vi "multi-rev.vi"(11 "设备信息":T2) -> ()   [LabVIEW 2020]
uses:
  <vilib>/Utility/NIReport.llb/Report Type.ctl
  <vilib>/Utility/NIReport.llb/Append Numeric Table to Report (wrap).vi
  <vilib>/Utility/NIReport.llb/Append Text Table to Report (wrap).vi
  <vilib>/Utility/NIReport.llb/NI_report.lvclass
  support/Message Queue/Message Queue.lvlib
  support/User Event - Stop/User Event - Stop.lvlib
  setup/support/rev_setup.lvlib
  rev_meas/rev_meas.lvlib
  bas_meas/bas_meas.lvlib
  <vilib>/Utility/NIReport.llb/NI_ReportGenerationCore.lvlib
panel:
  in  "新的测量":T1
  in  "calibration":T3
  in  "HWsetup":T4
  in  "EM设置":T5
  in  "开始":T6
  in  "停止":T7
  in  "退出":T8
  in  "测试类型":enum32{"空场当前结果", "放样后当前结果", "分析结果", "导出报告"}(radio)
  out "鼠标抓取值3":T9
  in  "选项卡控件":T10(tab)
  out "鼠标抓取值1":T9
  out "每通道声级":cluster{"声级大小":string, "dB":string}[](array[cluster])
  out "空场测量状态":T11
  in  "空场测试完成状态":T12
  in  "空场测试结果":T13
  out "空场混响频谱图":cluster{dbl[], "所有X坐标":dbl[]}[](graph)
  in  "saveT1":T14
  in  "空场当前结果":i32(listbox)
  in  "T1计数":u32
  in  "loadT1":bool
  in  "空场结果至Excel":bool
  in  "返回空场测试":bool
  in  "deletelineT1":bool
  in  "clearlistT1":bool
  in  "空场测试结果（T1）":i32(listbox)
  out "鼠标抓取值2":T9
  out "放样后每通道声级":cluster{"声级大小":string, "dB":string}[](array[cluster])
  out "放样后测量状态":T11
  in  "放样后测试完成状态":T12
  in  "放样后测试结果":T13
  in  "放入样品后当前结果":i32(listbox)
  out "放入样品后混响频谱图":cluster{dbl[], "所有X坐标":dbl[]}[](graph)
  in  "saveT2":T14
  in  "返回放样后测试":bool
  in  "放入样品后测试结果（T2）":i32(listbox)
  in  "clearlistT2":bool
  in  "deletelineT2":bool
  in  "放样结果至Excel":bool
  in  "loadT2":bool
  in  "T2计数":u32
  in  "ExportReport":T15
  in  "All results to Excel":T16
  out "吸声频谱图":cluster{dbl[], "所有X坐标":dbl[]}[](graph)
  in  "All results":i32(listbox)
  in  "analysis":T17
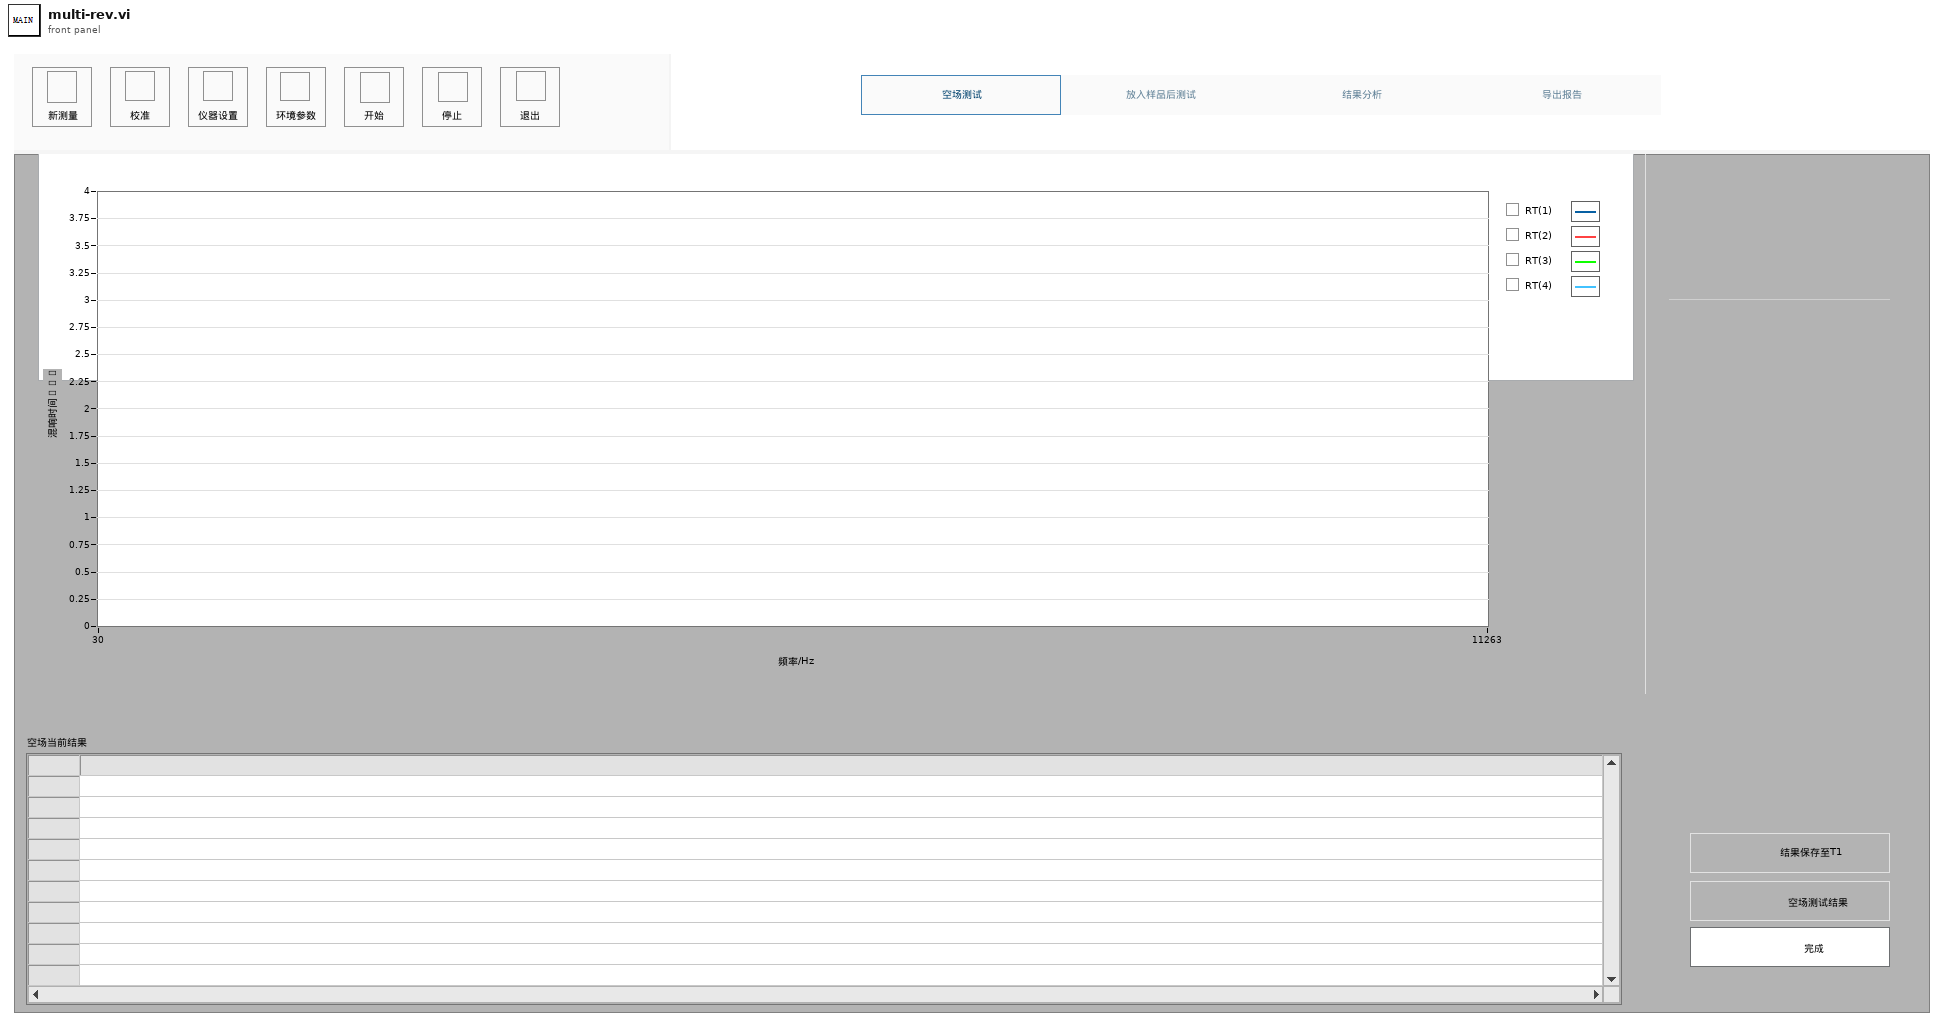
[diagram p1: front panel]
types:
  T1 = typedef "新测量.ctl" = bool
  T2 = cluster{"勾选的设备":refnum<visa-resource-name>[], "设备启用状态":cluster{"通道0":bool, "通道1":bool, "通道2":bool, "通道3":bool}}
  T3 = typedef "校准2.ctl" = bool
  T4 = typedef "硬件设置.ctl" = bool
  T5 = typedef "环境参数设置.ctl" = bool
  T6 = typedef "开始按钮.ctl" = bool
  T7 = typedef "停止按钮.ctl" = bool
  T8 = typedef "停止按钮2.ctl" = bool
  T9 = typedef "图谱移动字符串.ctl" = string
  T10 = enum32{"空场当前结果", "空场测试结果", "放入样品后当前结果", "放入样品后测试结果", "分析结果"}
  T11 = typedef "通道测量状态.ctl" = cluster{"通道编号":string, "通道测量状态":string}[]
  T12 = typedef "完成.ctl" = bool
  T13 = typedef "查看数据.ctl" = bool
  T14 = typedef "结果保存.ctl" = bool
  T15 = typedef "导出报表.ctl" = bool
  T16 = typedef "发送至Excel.ctl" = bool
  T17 = typedef "分析.ctl" = bool
  T18 = cluster{"通道编号输出":u32, "EDT":string, "T20":string, "T30":string}[]
  T19 = cluster{"空场当前结果":refnum<vi>, "放样后当前结果":refnum<vi>, "分析结果":refnum<vi>, "导出报告":refnum<vi>}
  T20 = typedef "Message Queue.lvlib/All Message Queues.ctl" = cluster{"UI":refnum<queue>, "采集":refnum<queue>, "记录":refnum<queue>}
  T21 = cluster{"T1":dbl[], "T2":dbl[], "A1":dbl[], "A2":dbl[], "AT":dbl[], "Aobj":dbl[], "αs":dbl[]}
  T22 = typedef "NI_ReportGenerationCore.lvlib/Report Type.ctl" = enum16{"HTML", "Word", "Excel"}
  T23 = cluster{"position (Excel)":cluster{"row":i32, "column":i32}, "name (Excel)":string, "bookmark (Word)":string}
  T24 = cluster{"T1":string[], "T2":string[], "A1":string[], "A2":string[], "AT":string[], "Aobj":string[], "αs":string[]}
  T25 = enum8{"Enabled", "Disabled", "Disabled and Grayed Out"}
  T26 = typedef "LVPoint32TypeDef.ctl" = cluster{"Horizontal":i32, "Vertical":i32}
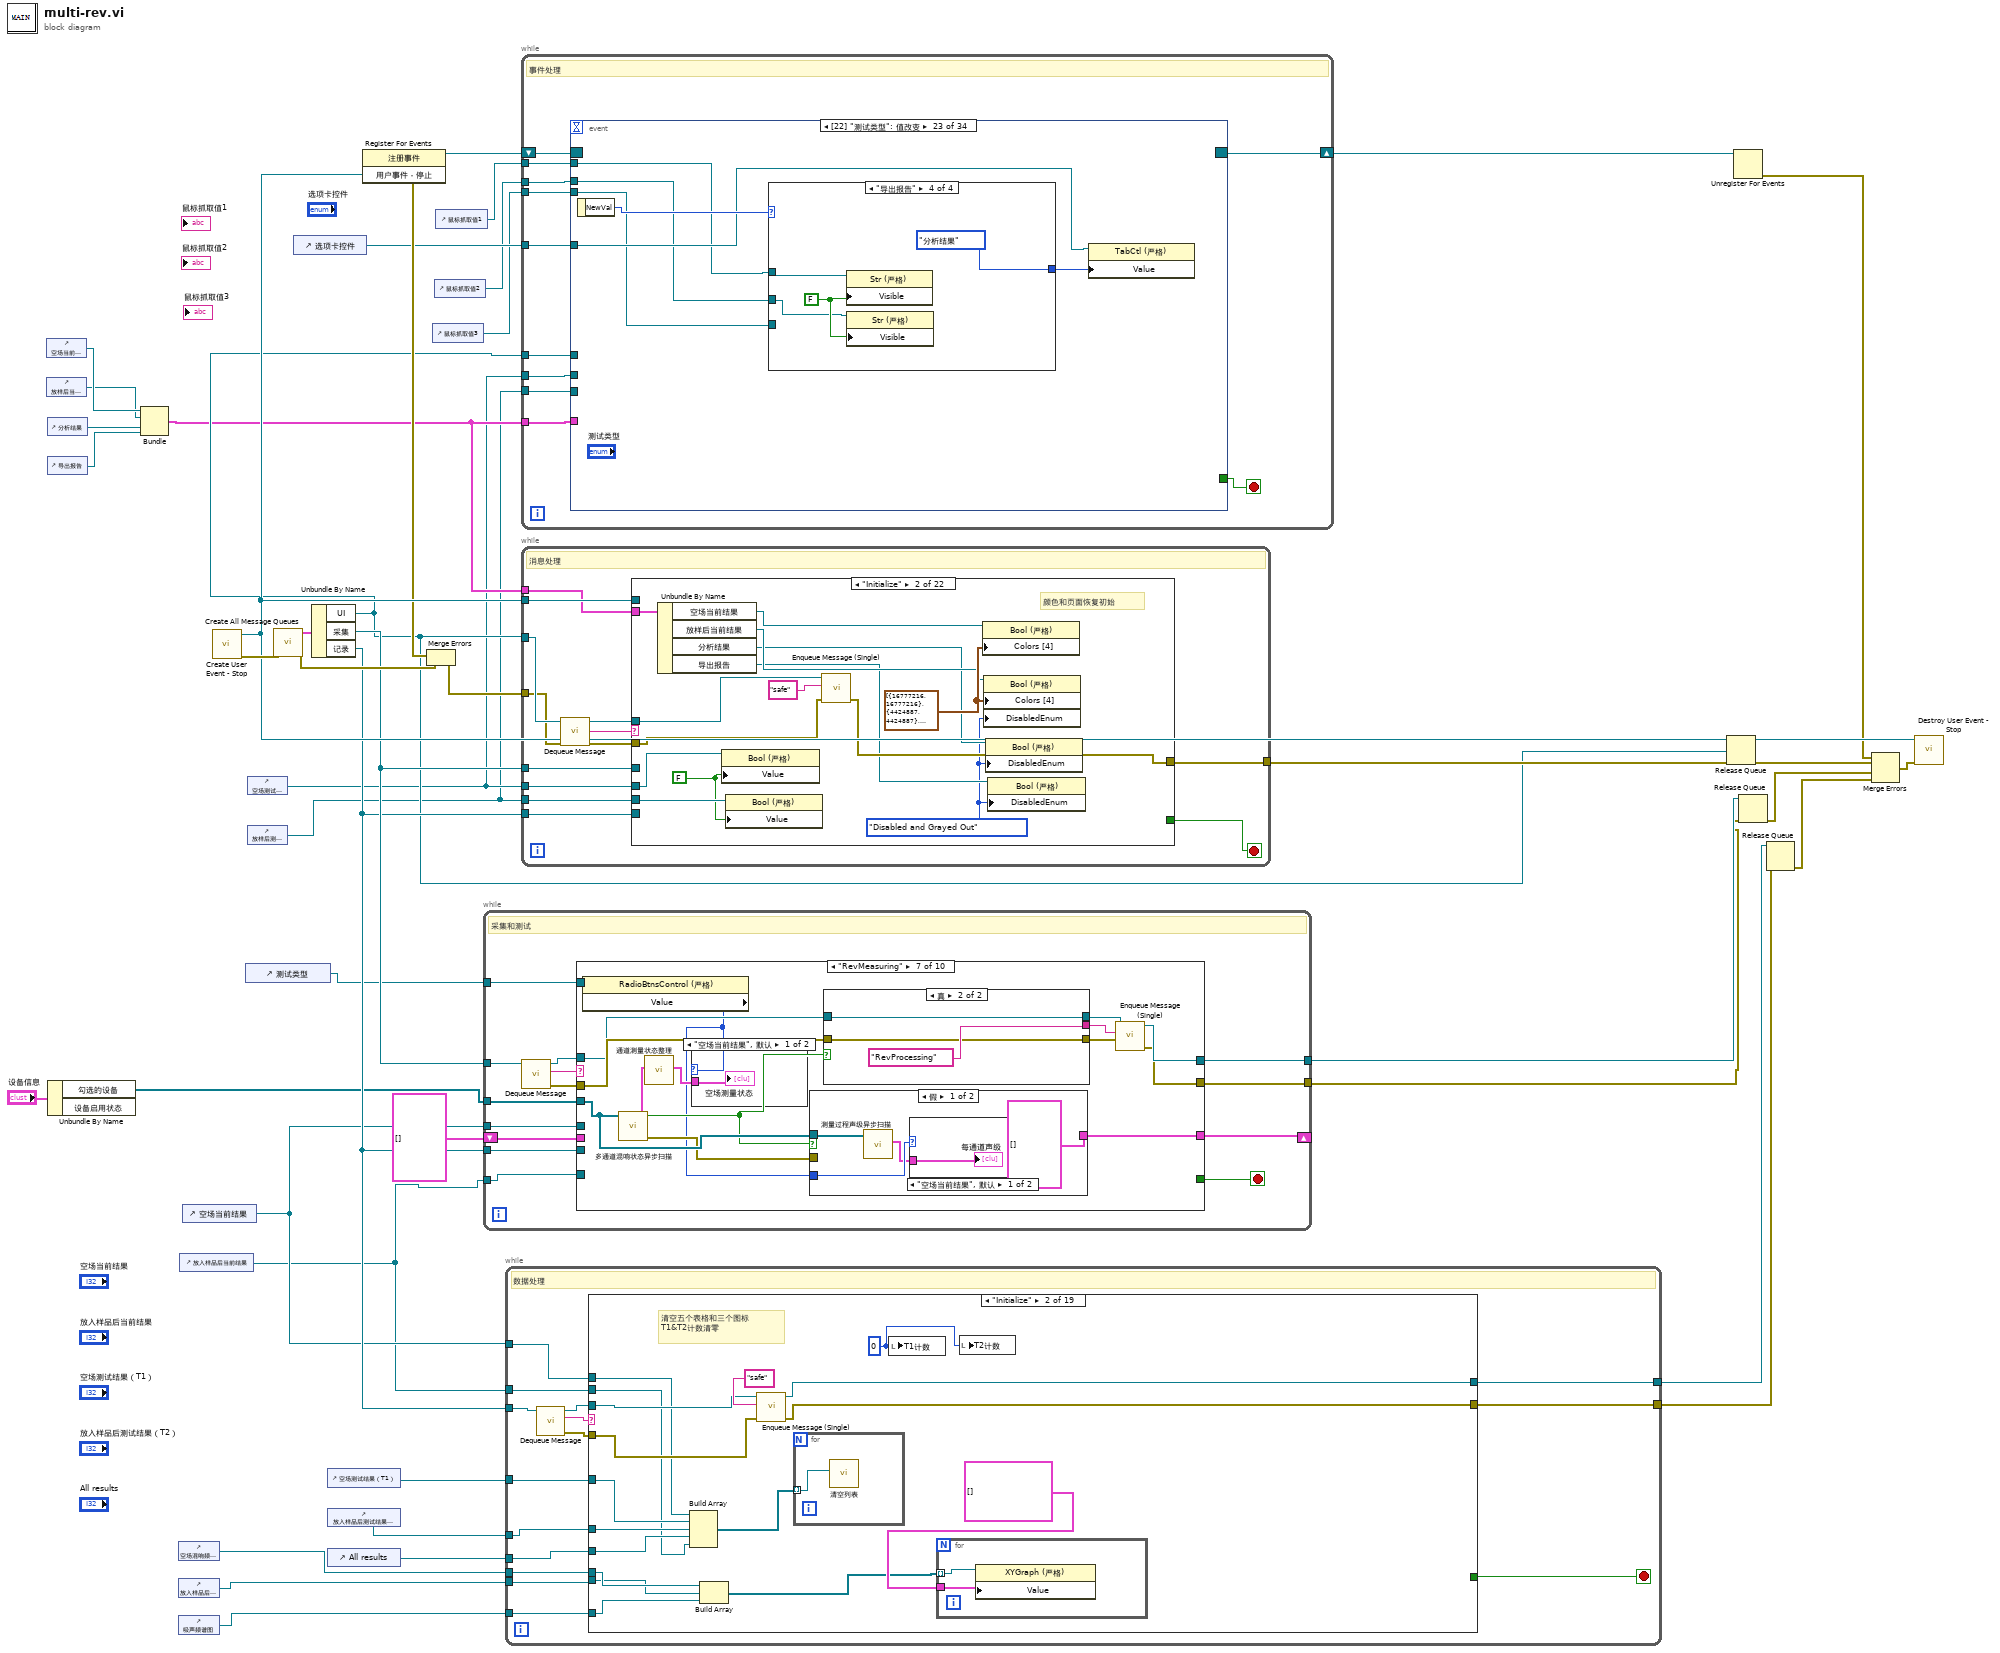
[diagram p0: block diagram]
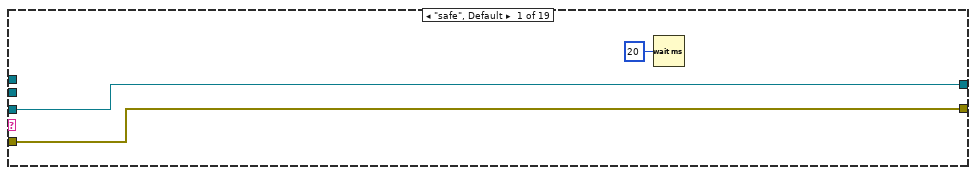
[diagram p2: hidden frame]
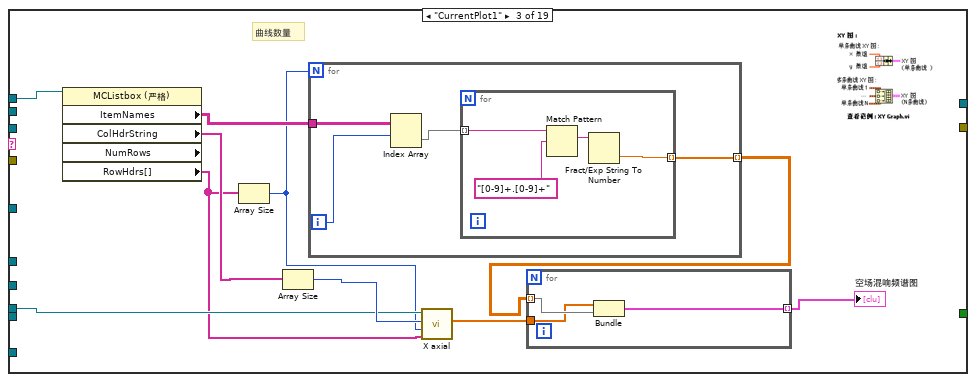
[diagram p3: hidden frame]
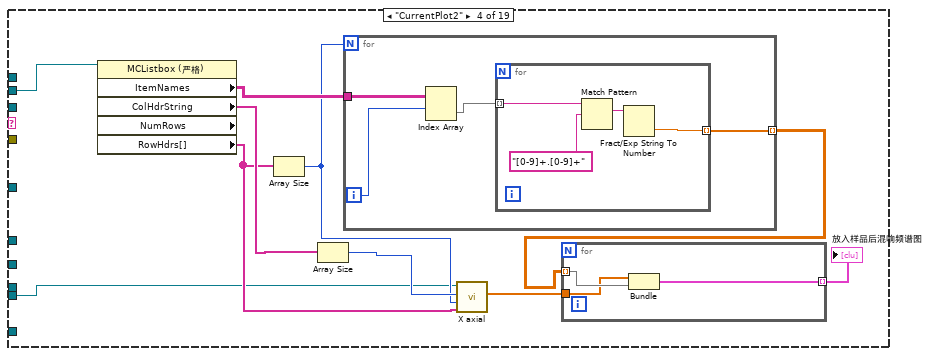
[diagram p4: hidden frame]
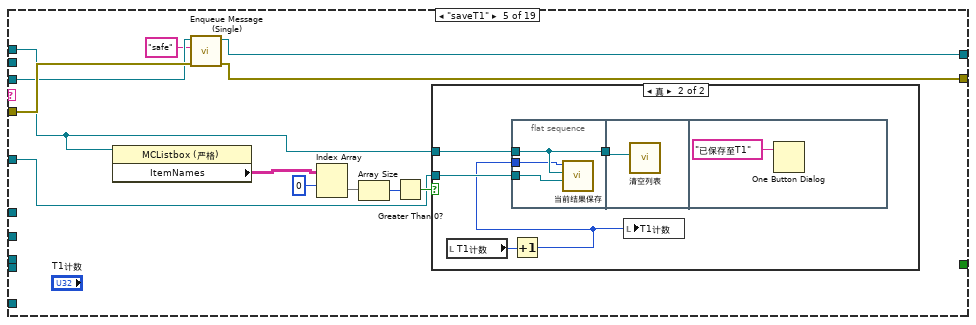
[diagram p5: hidden frame]
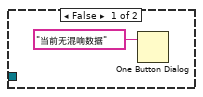
[diagram p6: hidden frame]
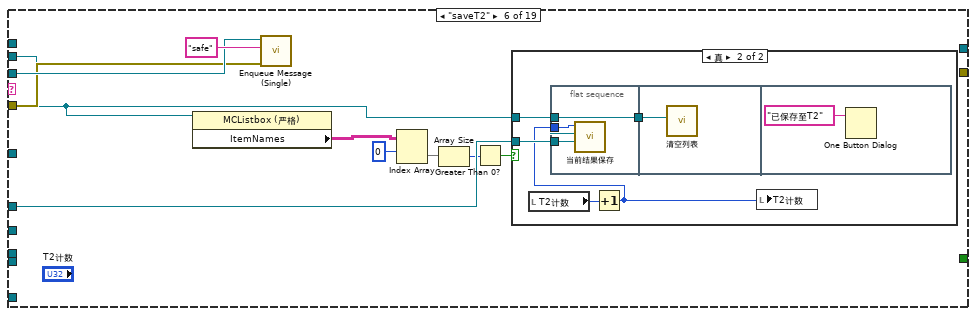
[diagram p7: hidden frame]
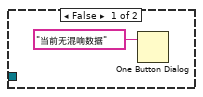
[diagram p8: hidden frame]
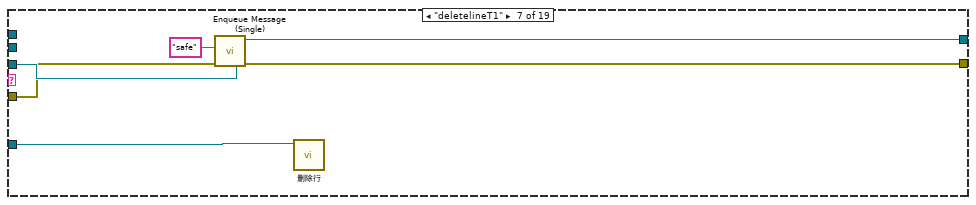
[diagram p9: hidden frame]
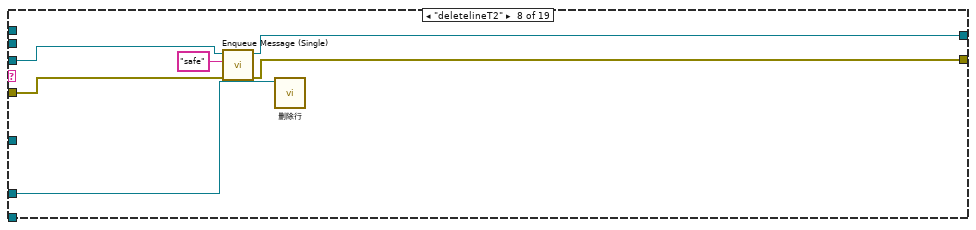
[diagram p10: hidden frame]
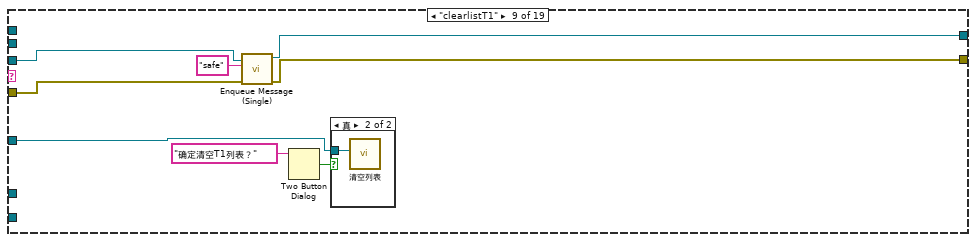
[diagram p11: hidden frame]
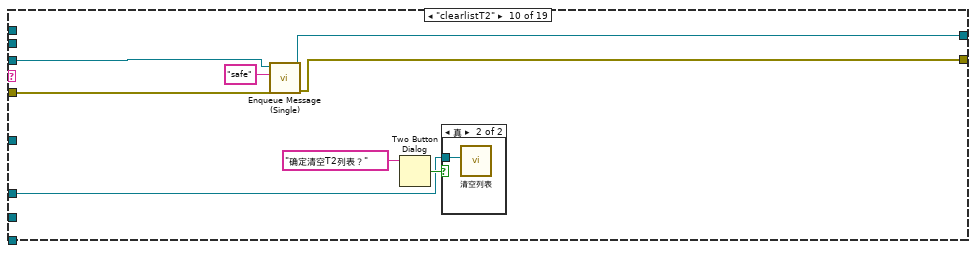
[diagram p13: hidden frame]
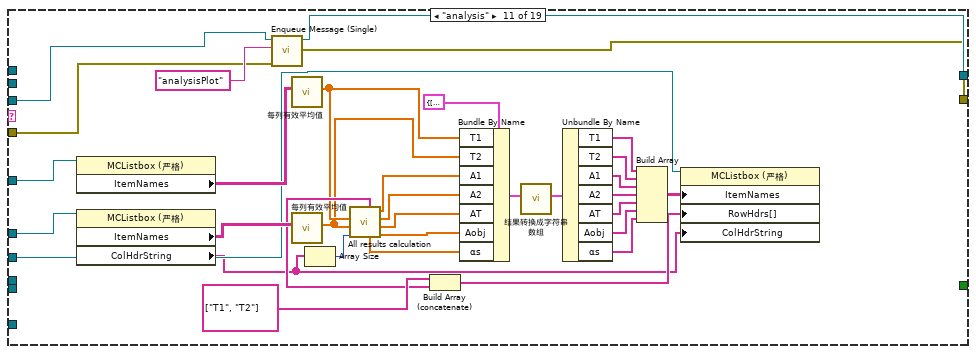
[diagram p15: hidden frame]
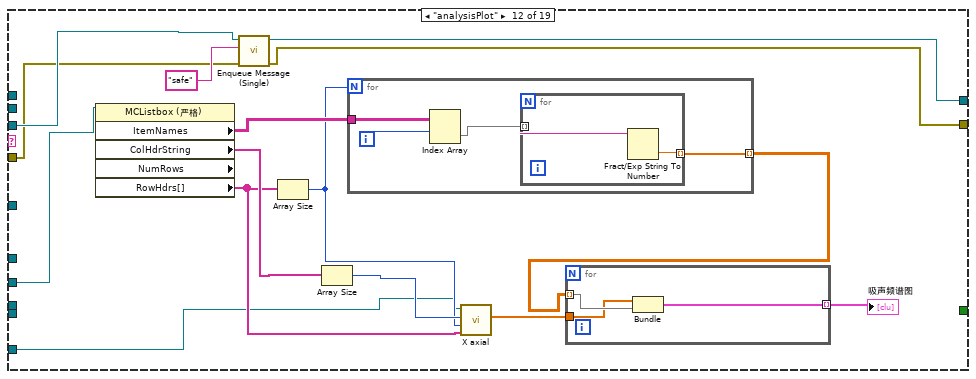
[diagram p16: hidden frame]
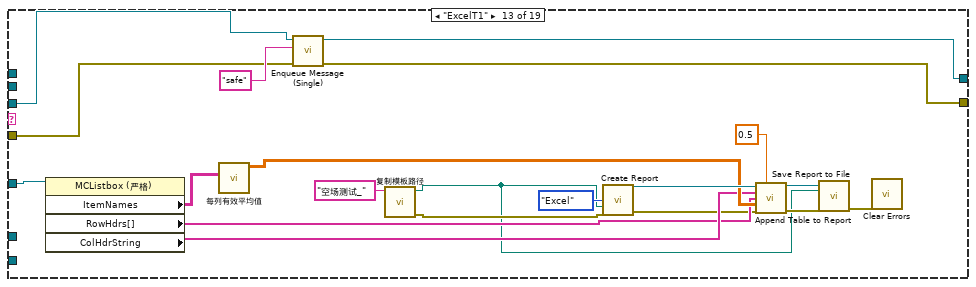
[diagram p17: hidden frame]
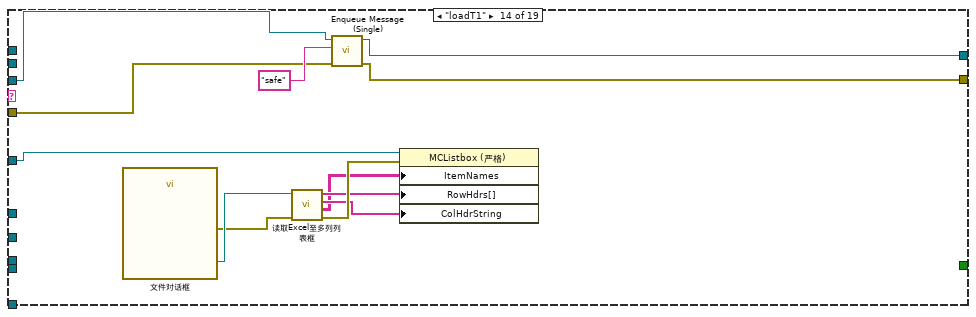
[diagram p18: hidden frame]
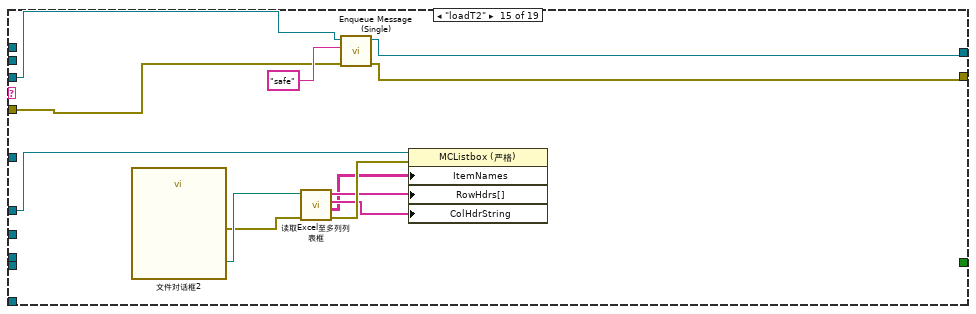
[diagram p19: hidden frame]
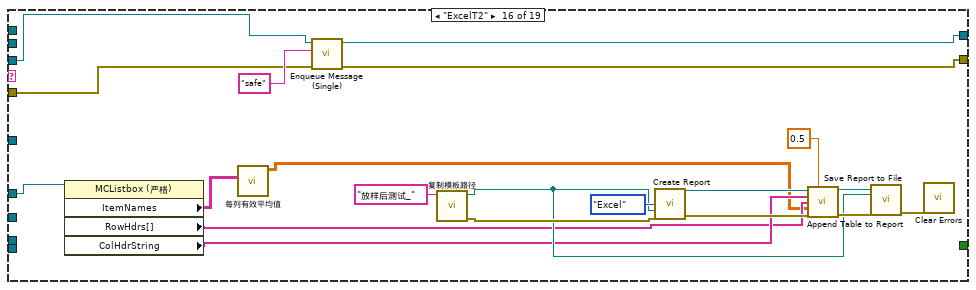
[diagram p20: hidden frame]
diagram:
  n1 = control-ref of="空场当前结果"() -> (w7:refnum<vi>)
  n2 = control-ref of="放样后当前结果"() -> (w6:refnum<vi>)
  n3 = control-ref of="分析结果"() -> (w5:refnum<vi>)
  n4 = control-ref of="导出报告"() -> (w4:refnum<vi>)
  n5 = Unbundle By Name("设备信息") -> ("勾选的设备"=w20:refnum<visa-resource-name>[])  [unwired: 1 out]
  n6 = Bundle("空场当前结果"=w7, "放样后当前结果"=w6, "分析结果"=w5, "导出报告"=w4) -> (w3:T19)  [unwired: 1 in]
  n7 = control-ref of="空场混响频谱图"() -> (w21:refnum<vi>)
  n8 = control-ref of="放入样品后混响频谱图"() -> (w14:refnum<vi>)
  n9 = control-ref of="吸声频谱图"() -> (w11:refnum<vi>)
  n10 = control-ref of="放入样品后当前结果"() -> (w15:refnum<vi>)
  n11 = control-ref of="空场当前结果"() -> (w17:refnum<vi>)
  n12 = call "Create User Event - Stop.vi"() -> ("error out"=w42:cluster{"状态":bool, "代码":i32, "源":string}, "用户事件－停止"=w41:refnum<user-event>)  [unwired: 10 in]
  n13 = control-ref of="测试类型"() -> (w12:refnum<vi>)
  n14 = control-ref of="空场测试完成状态"() -> (w2:refnum<vi>)
  n15 = control-ref of="放样后测试完成状态"() -> (w1:refnum<vi>)
  n16 = call "Create All Message Queues.vi"("error in (no error)"=w42) -> ("error out"=w39:cluster{"状态":bool, "代码":i32, "源":string}, "消息队列输出"=w44:T20)  [unwired: 9 in]
  n17 = control-ref of="选项卡控件"() -> (w13:refnum<vi>)
  n18 = Unbundle By Name(w44) -> ("UI"=w22:refnum<queue>, "采集"=w35:refnum<queue>, "记录"=w24:refnum<queue>)
  n19 = control-ref of="空场测试结果（T1）"() -> (w16:refnum<vi>)
  n20 = control-ref of="放入样品后测试结果（T2）"() -> (w25:refnum<vi>)
  n21 = control-ref of="All results"() -> (w23:refnum<vi>)
  n22 = register-events(w41) -> (reference out=w43:refnum<event-registration>, error out=w38:errorcluster)  [unwired: 2 in]
  n23 = Merge Errors(w38, w39) -> (w37:errorcluster)
  n24 = control-ref of="鼠标抓取值3"() -> (w8:refnum<vi>)
  n25 = control-ref of="鼠标抓取值2"() -> (w9:refnum<vi>)
  n26 = control-ref of="鼠标抓取值1"() -> (w10:refnum<vi>)
  n27 = while {
    tunnel: w35 -> [w58]
    tunnel: w17 -> [w53]
    tunnel: [w52] -> w31
    tunnel: [w51] -> w27
    tunnel: w24 -> [w50]
    shift-right: [w48] -> _
    shift-left: T18 [] ("所有混响RAW") -> [w47]
    tunnel: w20 -> [w49]
    tunnel: w15 -> [w46]
    tunnel: w12 -> [w45]
    stop <- w54 stop-if-true
    # "采集和测试"
    n28 = call "Dequeue Message.vi"("消息队列"=w58) -> ("error out"=w56:cluster{"状态":bool, "代码":i32, "源":string}, "消息"=w55:string, "消息队列副本"=w57:refnum<queue>)  [unwired: 7 in, 1 out]
    n29 = case shown="\"RevMeasuring\"" w55 {
      tunnel: w57 -> [_ w71 w79 w83 w89 w97 w116 w150 w166 w171]
      tunnel: w56 -> [_ w70 w80 _ w88 w96 w117 w149 w165 w169]
      tunnel: [_ _ _ _ _ _ _ _ _ TRUE] -> w54
      tunnel: w53 -> [_ _ _ _ _ _ _ w148 _ _]
      tunnel: [_ w69 w78 _ w87 w95 w112 _ _ w170] -> w52
      tunnel: [_ w68 w77 _ w86 w94 w111 w142 _ w168] -> w51
      tunnel: w50 -> [_ _ _ _ _ _ _ w146 _ _]
      tunnel: w49 -> [_ w67 _ _ w85 w99 w110 _ w164 _]
      tunnel: [w59 _ _ _ _ _ w107 _ _ _] -> w48
      tunnel: w47 -> [w59 _ _ _ _ _ _ w140 _ _]
      tunnel: w46 -> [_ _ _ _ _ _ _ w136 _ _]
      tunnel: w45 -> [_ _ _ _ _ _ w103 w135 _ _]
      frame "safe", Default {
        n30 = Wait (ms)(milliseconds to wait=u32 200 ("等待时间（毫秒）")) -> ()  [unwired: 1 out]
      }
      frame "Initialize" {
        # "首次运行初始化：恢复上一次设置"
        n31 = control-ref of="空场测量状态"() -> (w64:refnum<vi>)
        n32 = Array Size(array=w67) -> (size(s)=w65:i32)
        n33 = control-ref of="每通道声级"() -> (w63:refnum<vi>)
        n34 = call "rev-initialize.vi"("所有通道"=w67) -> ()  [unwired: 11 in]
        n35 = control-ref of="放样后测量状态"() -> (w62:refnum<vi>)
        n36 = control-ref of="放样后每通道声级"() -> (w61:refnum<vi>)
        n37 = call "Enqueue Message (Single).vi"("error in (no error)"=w70, "消息"="reInitialize", "消息队列"=w71) -> ("error out"=w68:cluster{"状态":bool, "代码":i32, "源":string}, "消息队列副本"=w69:refnum<queue>)  [unwired: 7 in]
        n38 = Build Array(w64, w62, w63, w61) -> (w66:refnum<vi>[])
        n39 = for {
          tunnel: w66 -> [w74] mode=indexing
          tunnel: w65 -> [w73]
          n40 = property class="Arr (严格)"(reference=w74, "Number of Rows"=w73) -> ()  [unwired: 1 in, 2 out]
        }
      }
      frame "reInitialize" {
        w76 = cluster{"声级大小":string, "dB":string}[] [{"声级大小"="---", "dB"=""}, {"声级大小"="---", "dB"=""}, {"声级大小"="---", "dB"=""}, {"声级大小"="---", "dB"=""}] ("每通道声级")
        w75 = cluster{"通道编号":string, "通道测量状态":string}[] [{"通道编号"="通道1：", "通道测量状态"="就绪..."}, {"通道编号"="通道2：", "通道测量状态"="就绪..."}, {"通道编号"="通道3", "通道测量状态"="就绪..."}, {"通道编号"="通道4", "通道测量状态"="就绪..."}] ("空场测量状态")
        n41 = local write "放样后每通道声级"(w76) -> ()
        n42 = local write "每通道声级"(w76) -> ()
        n43 = call "Enqueue Message (Single).vi"("error in (no error)"=w80, "消息"="safe", "消息队列"=w79) -> ("error out"=w77:cluster{"状态":bool, "代码":i32, "源":string}, "消息队列副本"=w78:refnum<queue>)  [unwired: 7 in]
        n44 = local write "空场测量状态"(w75) -> ()
        n45 = local write "放样后测量状态"(w75) -> ()
      }
      frame "calibration" {
        w82 = enum16{"通道1", "通道2", "通道3", "通道4"}."通道1" ("通道选择")
        n46 = call "Enqueue Message (Single).vi"("消息"="safe", "消息队列"=w83) -> ()  [unwired: 8 in, 2 out]
        n47 = call "SoundCalibration.vi"("通道号"=w82, "通道选择"=w82) -> ()  [unwired: 10 in]
      }
      frame "start" {
        n48 = for {
          tunnel: w85 -> [w92] mode=indexing
          n49 = VISA Write(VISA resource name=w92, write buffer="#1,S1;" ("写入缓冲区")) -> ()  [unwired: 1 in, 3 out]
          n50 = Wait (ms)(milliseconds to wait=u32 50 ("等待时间（毫秒）")) -> ()  [unwired: 1 out]
        }
        n51 = call "Enqueue Message (Single).vi"("error in (no error)"=w88, "消息"="RevMeasuring", "消息队列"=w89) -> ("error out"=w86:cluster{"状态":bool, "代码":i32, "源":string}, "消息队列副本"=w87:refnum<queue>)  [unwired: 7 in]
      }
      frame "stop" {
        n52 = call "Enqueue Message (Single).vi"("error in (no error)"=w96, "消息"="safe", "消息队列"=w97) -> ("error out"=w94:cluster{"状态":bool, "代码":i32, "源":string}, "消息队列副本"=w95:refnum<queue>)  [unwired: 7 in]
        n53 = for {
          tunnel: w99 -> [w101] mode=indexing
          n54 = VISA Write(VISA resource name=w101, write buffer="#1,S0;" ("写入缓冲区")) -> ()  [unwired: 1 in, 3 out]
          n55 = Wait (ms)(milliseconds to wait=u32 50 ("等待时间（毫秒）")) -> ()  [unwired: 1 out]
        }
      }
      frame "RevMeasuring" {
        n56 = property class="RadioBtnsControl (严格)"(reference=w103) -> ("Value"=w104:enum32{"空场当前结果", "放样后当前结果", "分析结果", "导出报告"})  [unwired: 1 in, 2 out]
        n57 = call "多通道混响状态异步扫描.vi"("勾选的设备"=w110) -> ("error out"=w109:errorcluster, "所有测量状态"=w106:cluster{"通道编号输出":u32, "测量状态":string}[], "所有测量是否完成？"=w108:bool)  [unwired: 8 in]
        n58 = call "通道测量状态整理.vi"("所有测量状态"=w106) -> ("所有通道状态"=w105:cluster{"通道号":string, "通道测量状态":string}[])  [unwired: 10 in]
        n59 = case shown="\"空场当前结果\", 默认" w104 {
          tunnel: w105 -> [w118 w119]
          frame "空场当前结果", Default {
            "空场测量状态" <- w118
          }
          frame "放样后当前结果" {
            "放样后测量状态" <- w119
          }
        }
        n60 = case shown="假" w108 {
          tunnel: w110 -> [w122 w128]
          tunnel: w109 -> [_ w127]
          tunnel: [T18 [] ("所有混响RAW") w126] -> w107
          tunnel: w104 -> [w121 _]
          frame False {
            n61 = call "测量过程声级异步扫描.vi"("设备选择"=w122) -> ("每通道声级"=w120:cluster{"字符串":string, "dB字符":string}[])  [unwired: 10 in]
            n62 = case shown="\"空场当前结果\", 默认" w121 {
              tunnel: w120 -> [w124 w125]
              frame "空场当前结果", Default {
                "每通道声级" <- w124
              }
              frame "放样后当前结果" {
                "放样后每通道声级" <- w125
              }
            }
          }
          frame True {
            n63 = call "多通道混响数据异步获取.vi"("错误输入（无错误） 2"=w127, "勾选的设备 2"=w128) -> ("所有通道混响RAW"=w126:T18)  [unwired: 8 in, 1 out]
          }
        }
        n64 = case shown="真" w108 {
          tunnel: w117 -> [w129 w132]
          tunnel: w116 -> [w130 w133]
          tunnel: ["RevMeasuring" ("消息") "RevProcessing" ("消息")] -> w115
          tunnel: [w130 w133] -> w114
          tunnel: [w129 w132] -> w113
          frame False {
          }
          frame True {
          }
        }
        n65 = call "Enqueue Message (Single).vi"("error in (no error)"=w113, "消息"=w115, "消息队列"=w114) -> ("error out"=w111:cluster{"状态":bool, "代码":i32, "源":string}, "消息队列副本"=w112:refnum<queue>)  [unwired: 7 in]
      }
      frame "RevProcessing" {
        # "FRE\nEDT\nT20\nT30\nRT"
        n66 = property class="RadioBtnsControl (严格)"(reference=w135) -> ("Value"=w137:enum32{"空场当前结果", "放样后当前结果", "分析结果", "导出报告"})  [unwired: 1 in, 2 out]
        n67 = call "多通道混响数据处理.vi"("所有混响RAW"=w140) -> ("所有RT混响数据"=w139:string[][], "频率输出"=w141:string[], "所有RT行首"=w138:string[])  [unwired: 6 in, 2 out]
        n68 = call "Enqueue Message (Single).vi"("error in (no error)"=w149, "消息"="safe", "消息队列"=w150) -> ("error out"=w144:cluster{"状态":bool, "代码":i32, "源":string})  [unwired: 7 in, 1 out]
        n69 = case shown="\"空场当前结果\", 默认" w137 {
          tunnel: w148 -> [w157 _]
          tunnel: ["CurrentPlot1" ("消息") "CurrentPlot2" ("消息")] -> w147
          tunnel: [w153 w162] -> w145
          tunnel: w141 -> [w155 w161]
          tunnel: w139 -> [w156 w160]
          tunnel: w138 -> [w154 w159]
          tunnel: w136 -> [_ w158]
          frame "空场当前结果", Default {
            n70 = property class="MCListbox (严格)"(reference=w157, "ItemNames"=w156, "ColHdrString"=w155, "RowHdrs[]"=w154) -> (error out=w153:errorcluster)  [unwired: 1 in, 1 out]
          }
          frame "放样后当前结果" {
            n71 = property class="MCListbox (严格)"(reference=w158, "ItemNames"=w160, "ColHdrString"=w161, "RowHdrs[]"=w159) -> (error out=w162:errorcluster)  [unwired: 1 in, 1 out]
          }
        }
        n72 = call "Enqueue Message (Single).vi"("error in (no error)"=w145, "消息"=w147, "消息队列"=w146) -> ("error out"=w143:cluster{"状态":bool, "代码":i32, "源":string})  [unwired: 7 in, 1 out]
        n73 = Merge Errors(w144, w143) -> (w142:errorcluster)
      }
      frame "HWsetup" {
        n74 = call "HWsetup options.vi"("所有通道"=w164) -> ()  [unwired: 11 in]
        n75 = call "Enqueue Message (Single).vi"("error in (no error)"=w165, "消息"="safe", "消息队列"=w166) -> ()  [unwired: 7 in, 2 out]
      }
      frame "Exti" {
        n76 = Flush Queue(queue=w171, error in (no error)=w169) -> (queue out=w170:refnum<queue>, error out=w168:errorcluster)  [unwired: 1 out]
      }
    }
  }
  n77 = while {
    tunnel: w24 -> [w186]
    tunnel: w17 -> [w184]
    tunnel: [w181] -> w29
    tunnel: [w180] -> w26
    tunnel: w16 -> [w179]
    tunnel: w25 -> [w178]
    tunnel: w23 -> [w177]
    tunnel: w21 -> [w176]
    tunnel: w15 -> [w175]
    tunnel: w14 -> [w174]
    tunnel: w11 -> [w173]
    stop <- w185 stop-if-true
    # "数据处理"
    n78 = call "Dequeue Message.vi"("消息队列"=w186) -> ("error out"=w182:cluster{"状态":bool, "代码":i32, "源":string}, "消息"=w187:string, "消息队列副本"=w183:refnum<queue>)  [unwired: 7 in, 1 out]
    n79 = case shown="\"Initialize\"" w187 {
      tunnel: [_ _ _ _ _ _ _ _ _ _ _ _ _ _ _ _ _ _ TRUE] -> w185
      tunnel: w184 -> [_ w204 w220 _ w254 _ _ _ _ _ _ _ _ _ _ _ _ _ _]
      tunnel: w183 -> [w189 w206 _ _ w261 w284 w301 w307 w313 w321 w358 w365 w402 w407 w418 w444 w464 w478 w491]
      tunnel: w182 -> [w188 w205 _ _ w264 w283 w300 w306 w312 w322 w357 w364 w401 w406 w417 w445 w463 w477 w489]
      tunnel: [w189 w198 _ _ w263 _ w299 w305 w315 w324 w356 w363 w400 w405 w420 w443 _ _ w490] -> w181
      tunnel: [w188 w197 _ _ w262 _ w298 w304 w314 w323 w355 w362 w399 w404 w419 w442 _ _ w488] -> w180
      tunnel: w179 -> [_ w203 _ _ w255 _ w297 _ w309 _ w354 _ w398 w414 _ _ _ _ _]
      tunnel: w178 -> [_ w202 _ _ _ w282 _ w303 _ w318 w353 _ _ _ w416 w441 _ _ _]
      tunnel: w177 -> [_ w201 _ _ _ _ _ _ _ _ w350 w367 _ _ _ _ w462 w476 _]
      tunnel: w176 -> [_ w196 w213 _ _ _ _ _ _ _ _ _ _ _ _ _ _ _ _]
      tunnel: w175 -> [_ w199 _ w234 _ w276 _ _ _ _ _ _ _ _ _ _ _ _ _]
      tunnel: w174 -> [_ w195 _ w233 _ _ _ _ _ _ _ _ _ _ _ _ _ _ _]
      tunnel: w173 -> [_ w194 _ _ _ _ _ _ _ _ _ w360 _ _ _ _ _ w472 _]
      frame "safe", Default {
        n80 = Wait (ms)(milliseconds to wait=u32 20 ("等待时间（毫秒）")) -> ()  [unwired: 1 out]
      }
      frame "Initialize" {
        w191 = u32 0 ("T1计数")
        # "清空五个表格和三个图标\nT1&T2计数清零"
        n81 = Build Array(w204, w203, w202, w201, w199) -> (w200:refnum<vi>[])
        n82 = Build Array(w196, w195, w194) -> (w192:refnum<vi>[])
        n83 = call "Enqueue Message (Single).vi"("error in (no error)"=w205, "消息"="safe", "消息队列"=w206) -> ("error out"=w197:cluster{"状态":bool, "代码":i32, "源":string}, "消息队列副本"=w198:refnum<queue>)  [unwired: 7 in]
        n84 = for {
          tunnel: w200 -> [w210] mode=indexing
          n85 = call "清空列表.vi"("列表"=w210) -> ()  [unwired: 11 in]
        }
        n86 = local write "T1计数"(w191) -> ()
        n87 = for {
          tunnel: cluster{dbl[], "所有X坐标":dbl[]}[] [] ("值") -> [w208]
          tunnel: w192 -> [w209] mode=indexing
          n88 = property class="XYGraph (严格)"(reference=w209, "Value"=w208) -> ()  [unwired: 1 in, 2 out]
        }
        n89 = local write "T2计数"(w191) -> ()
      }
      frame "CurrentPlot1" {
        # "曲线数量"
        n90 = property class="MCListbox (严格)" props=["ItemNames", "ColHdrString", "NumRows", "RowHdrs[]"](reference=w220) -> ("ItemNames"=w217:string[][], "ColHdrString"=w218:string[], "RowHdrs[]"=w212:string[])  [unwired: 1 in, 3 out]
        n91 = Array Size(array=w212) -> (size(s)=w211:i32)
        n92 = Array Size(array=w218) -> (size(s)=w219:i32)
        n93 = for {
          N: w211 -> [_]
          tunnel: [w227] -> w216 mode=indexing
          tunnel: w217 -> [w226]
          i -> [w224]
          n94 = Index Array(array=w226, index (row)=w224) -> (element=w225:string[])  [unwired: 1 in]
          n95 = for {
            tunnel: [w229] -> w227 mode=indexing
            tunnel: w225 -> [w228] mode=indexing
            n96 = Match Pattern(string=w228, regular expression="[0-9]+.[0-9]+" ("正则表达式")) -> (match substring=w230:string)  [unwired: 1 in, 3 out]
            n97 = Fract/Exp String To Number(string=w230) -> (number=w229:dbl)  [unwired: 3 in, 1 out]
          }
        }
        n98 = call "X axial.vi"("曲线名称"=w212, "曲线数量"=w211, "频率配置"=w219, "当前混响频谱图"=w213) -> ("所有X坐标"=w215:dbl[])  [unwired: 7 in]
        n99 = for {
          tunnel: w216 -> [w222] mode=indexing
          tunnel: w215 -> [w221]
          tunnel: [w223] -> w214 mode=indexing
          n100 = Bundle("所有X坐标"=w221, w222) -> (w223:cluster{"所有X坐标":dbl[], dbl[]})  [unwired: 1 in]
        }
        "空场混响频谱图" <- w214
      }
      frame "CurrentPlot2" {
        n101 = property class="MCListbox (严格)" props=["ItemNames", "ColHdrString", "NumRows", "RowHdrs[]"](reference=w234) -> ("ItemNames"=w239:string[][], "ColHdrString"=w240:string[], "RowHdrs[]"=w236:string[])  [unwired: 1 in, 3 out]
        n102 = Array Size(array=w236) -> (size(s)=w235:i32)
        n103 = Array Size(array=w240) -> (size(s)=w241:i32)
        n104 = for {
          N: w235 -> [_]
          tunnel: [w248] -> w238 mode=indexing
          tunnel: w239 -> [w247]
          i -> [w245]
          n105 = Index Array(array=w247, index (row)=w245) -> (element=w246:string[])  [unwired: 1 in]
          n106 = for {
            tunnel: [w250] -> w248 mode=indexing
            tunnel: w246 -> [w249] mode=indexing
            n107 = Match Pattern(string=w249, regular expression="[0-9]+.[0-9]+" ("正则表达式")) -> (match substring=w251:string)  [unwired: 1 in, 3 out]
            n108 = Fract/Exp String To Number(string=w251) -> (number=w250:dbl)  [unwired: 3 in, 1 out]
          }
        }
        n109 = call "X axial.vi"("曲线名称"=w236, "曲线数量"=w235, "频率配置"=w241, "当前混响频谱图"=w233) -> ("所有X坐标"=w237:dbl[])  [unwired: 7 in]
        n110 = for {
          tunnel: w238 -> [w243] mode=indexing
          tunnel: w237 -> [w242]
          tunnel: [w244] -> w232 mode=indexing
          n111 = Bundle("所有X坐标"=w242, w243) -> (w244:cluster{"所有X坐标":dbl[], dbl[]})  [unwired: 1 in]
        }
        "放入样品后混响频谱图" <- w232
      }
      frame "saveT1" {
        n112 = property class="MCListbox (严格)"(reference=w254) -> ("ItemNames"=w259:string[][])  [unwired: 1 in, 2 out]
        n113 = call "Enqueue Message (Single).vi"("error in (no error)"=w264, "消息"="safe", "消息队列"=w261) -> ("error out"=w262:cluster{"状态":bool, "代码":i32, "源":string}, "消息队列副本"=w263:refnum<queue>)  [unwired: 7 in]
        n114 = Index Array(array=w259, index (row)=0 ("索引 (行)")) -> (element=w257:string[])  [unwired: 1 in]
        n115 = Array Size(array=w257) -> (size(s)=w260:i32)
        n116 = Greater Than 0?(x=w260) -> (x > 0?=w256:bool)
        n117 = case shown="真" w256 {
          tunnel: w255 -> [_ w270]
          tunnel: w254 -> [_ w269]
          frame False {
            n118 = One Button Dialog(message="当前无混响数据" ("消息")) -> ()  [unwired: 1 in, 1 out]
          }
          frame True {
            n119 = local read "T1计数"() -> (w267:u32)
            n120 = flat-sequence {
              tunnel: w270 -> [w273]
              tunnel: w269 -> [w272]
              tunnel: [w272] -> w268
              tunnel: w266 -> [w271]
              tunnel: w268 -> [w274]
              frame #0 {
                n121 = call "当前结果保存.vi"("列表2"=w273, "列表1"=w272, "保存计数"=w271) -> ()  [unwired: 9 in]
              }
              frame #1 {
                n122 = call "清空列表.vi"("列表"=w274) -> ()  [unwired: 11 in]
              }
              frame #2 {
                n123 = One Button Dialog(message="已保存至T1" ("消息")) -> ()  [unwired: 1 in, 1 out]
              }
            }
            n124 = Increment(x=w267) -> (x+1=w266:u32)
            n125 = local write "T1计数"(w266) -> ()
          }
        }
      }
      frame "saveT2" {
        n126 = property class="MCListbox (严格)"(reference=w276) -> ("ItemNames"=w280:string[][])  [unwired: 1 in, 2 out]
        n127 = call "Enqueue Message (Single).vi"("error in (no error)"=w283, "消息"="safe", "消息队列"=w284) -> ()  [unwired: 7 in, 2 out]
        n128 = Index Array(array=w280, index (row)=0 ("索引 (行)")) -> (element=w278:string[])  [unwired: 1 in]
        n129 = Array Size(array=w278) -> (size(s)=w281:i32)
        n130 = Greater Than 0?(x=w281) -> (x > 0?=w277:bool)
        n131 = case shown="真" w277 {
          tunnel: w282 -> [_ w291]
          tunnel: w276 -> [_ w290]
          frame False {
            n132 = One Button Dialog(message="当前无混响数据" ("消息")) -> ()  [unwired: 1 in, 1 out]
          }
          frame True {
            n133 = local read "T2计数"() -> (w288:u32)
            n134 = flat-sequence {
              tunnel: w291 -> [w294]
              tunnel: w290 -> [w293]
              tunnel: [w293] -> w289
              tunnel: w287 -> [w292]
              tunnel: w289 -> [w295]
              frame #0 {
                n135 = call "当前结果保存.vi"("列表2"=w294, "列表1"=w293, "保存计数"=w292) -> ()  [unwired: 9 in]
              }
              frame #1 {
                n136 = call "清空列表.vi"("列表"=w295) -> ()  [unwired: 11 in]
              }
              frame #2 {
                n137 = One Button Dialog(message="已保存至T2" ("消息")) -> ()  [unwired: 1 in, 1 out]
              }
            }
            n138 = Increment(x=w288) -> (x+1=w287:u32)
            n139 = local write "T2计数"(w287) -> ()
          }
        }
      }
      frame "deletelineT1" {
        n140 = call "Enqueue Message (Single).vi"("error in (no error)"=w300, "消息"="safe", "消息队列"=w301) -> ("error out"=w298:cluster{"状态":bool, "代码":i32, "源":string}, "消息队列副本"=w299:refnum<queue>)  [unwired: 7 in]
        n141 = call "删除行.vi"("列表"=w297) -> ()  [unwired: 11 in]
      }
      frame "deletelineT2" {
        n142 = call "Enqueue Message (Single).vi"("error in (no error)"=w306, "消息"="safe", "消息队列"=w307) -> ("error out"=w304:cluster{"状态":bool, "代码":i32, "源":string}, "消息队列副本"=w305:refnum<queue>)  [unwired: 7 in]
        n143 = call "删除行.vi"("列表"=w303) -> ()  [unwired: 11 in]
      }
      frame "clearlistT1" {
        n144 = call "Enqueue Message (Single).vi"("error in (no error)"=w312, "消息"="safe", "消息队列"=w313) -> ("error out"=w314:cluster{"状态":bool, "代码":i32, "源":string}, "消息队列副本"=w315:refnum<queue>)  [unwired: 7 in]
        n145 = Two Button Dialog(message="确定清空T1列表？" ("消息")) -> (T button?=w310:bool)  [unwired: 2 in]
        n146 = case shown="真" w310 {
          tunnel: w309 -> [_ w317]
          frame False {
          }
          frame True {
            n147 = call "清空列表.vi"("列表"=w317) -> ()  [unwired: 11 in]
          }
        }
      }
      frame "clearlistT2" {
        n148 = call "Enqueue Message (Single).vi"("error in (no error)"=w322, "消息"="safe", "消息队列"=w321) -> ("error out"=w323:cluster{"状态":bool, "代码":i32, "源":string}, "消息队列副本"=w324:refnum<queue>)  [unwired: 7 in]
        n149 = Two Button Dialog(message="确定清空T2列表？" ("消息")) -> (T button?=w319:bool)  [unwired: 2 in]
        n150 = case shown="真" w319 {
          tunnel: w318 -> [_ w326]
          frame False {
          }
          frame True {
            n151 = call "清空列表.vi"("列表"=w326) -> ()  [unwired: 11 in]
          }
        }
      }
      frame "analysis" {
        n152 = property class="MCListbox (严格)"(reference=w354) -> ("ItemNames"=w352:string[][])  [unwired: 1 in, 2 out]
        n153 = property class="MCListbox (严格)"(reference=w353) -> ("ItemNames"=w351:string[][], "ColHdrString"=w328:string[])  [unwired: 1 in, 2 out]
        n154 = call "Enqueue Message (Single).vi"("error in (no error)"=w357, "消息"="analysisPlot", "消息队列"=w358) -> ("error out"=w355:cluster{"状态":bool, "代码":i32, "源":string}, "消息队列副本"=w356:refnum<queue>)  [unwired: 7 in]
        n155 = call "每列有效平均值.vi"("测试数组"=w352) -> ("平均混响时间"=w346:dbl[])  [unwired: 9 in, 1 out]
        n156 = call "每列有效平均值.vi"("测试数组"=w351) -> ("平均混响时间"=w345:dbl[])  [unwired: 9 in, 1 out]
        n157 = Array Size(array=w328) -> (size(s)=w327:i32)
        n158 = call "All results calculation.vi"("频率配置"=w327, "平均混响时间T2"=w345, "平均混响时间T1"=w346) -> ("分立吸声体吸声量Aobj"=w341:dbl[], "试件吸声量AT"=w342:dbl[], "混响室吸声量A2"=w343:dbl[], "混响室吸声量A1"=w344:dbl[], "吸声系数αs"=w340:dbl[], "rowhead"=w348:string[])  [unwired: 3 in]
        n159 = Build Array (concatenate)(string[] ["T1", "T2"], w348) -> (w329:string[])
        n160 = Bundle By Name(cluster=T21 {"T1"=[], "T2"=[], "A1"=[], "A2"=[], "AT"=[], "Aobj"=[], "αs"=[]} ("结果数据数组簇"), "T1"=w346, "T2"=w345, "A1"=w344, "A2"=w343, "AT"=w342, "Aobj"=w341, "αs"=w340) -> (w339:T21)
        n161 = call "结果转换成字符串数组.vi"("结果数据数组簇"=w339) -> ("结果字符串数组簇"=w338:T24)  [unwired: 10 in]
        n162 = Unbundle By Name(w338) -> ("T1"=w337:string[], "T2"=w336:string[], "A1"=w335:string[], "A2"=w334:string[], "AT"=w333:string[], "Aobj"=w332:string[], "αs"=w331:string[])
        n163 = Build Array(w337, w336, w335, w334, w333, w332, w331) -> (w330:string[][])
        n164 = property class="MCListbox (严格)"(reference=w350, "ItemNames"=w330, "RowHdrs[]"=w329, "ColHdrString"=w328) -> ()  [unwired: 1 in, 2 out]
      }
      frame "analysisPlot" {
        n165 = property class="MCListbox (严格)" props=["ItemNames", "ColHdrString", "NumRows", "RowHdrs[]"](reference=w367) -> ("ItemNames"=w372:string[][], "ColHdrString"=w373:string[], "RowHdrs[]"=w369:string[])  [unwired: 1 in, 3 out]
        n166 = call "Enqueue Message (Single).vi"("error in (no error)"=w364, "消息"="safe", "消息队列"=w365) -> ("error out"=w362:cluster{"状态":bool, "代码":i32, "源":string}, "消息队列副本"=w363:refnum<queue>)  [unwired: 7 in]
        n167 = Array Size(array=w369) -> (size(s)=w368:i32)
        n168 = Array Size(array=w373) -> (size(s)=w374:i32)
        n169 = for {
          N: w368 -> [_]
          tunnel: [w381] -> w371 mode=indexing
          tunnel: w372 -> [w380]
          i -> [w378]
          n170 = Index Array(array=w380, index (row)=w378) -> (element=w379:string[])  [unwired: 1 in]
          n171 = for {
            tunnel: [w383] -> w381 mode=indexing
            tunnel: w379 -> [w382] mode=indexing
            n172 = Fract/Exp String To Number(string=w382) -> (number=w383:dbl)  [unwired: 3 in, 1 out]
          }
        }
        n173 = call "X axial.vi"("曲线名称"=w369, "曲线数量"=w368, "频率配置"=w374, "当前混响频谱图"=w360) -> ("所有X坐标"=w370:dbl[])  [unwired: 7 in]
        n174 = for {
          tunnel: w371 -> [w376] mode=indexing
          tunnel: w370 -> [w375]
          tunnel: [w377] -> w361 mode=indexing
          n175 = Bundle("所有X坐标"=w375, w376) -> (w377:cluster{"所有X坐标":dbl[], dbl[]})  [unwired: 1 in]
        }
        "吸声频谱图" <- w361
      }
      frame "ExcelT1" {
        n176 = property class="MCListbox (严格)"(reference=w398) -> ("ItemNames"=w397:string[][], "RowHdrs[]"=w392:string[], "ColHdrString"=w393:string[])  [unwired: 1 in, 2 out]
        n177 = call "每列有效平均值.vi"("测试数组"=w397) -> ("混响2D数值"=w394:dbl[][])  [unwired: 9 in, 1 out]
        n178 = call "Enqueue Message (Single).vi"("error in (no error)"=w401, "消息"="safe", "消息队列"=w402) -> ("error out"=w399:cluster{"状态":bool, "代码":i32, "源":string}, "消息队列副本"=w400:refnum<queue>)  [unwired: 7 in]
        n179 = call "复制模板路径.vi"("名称前缀"="空场测试_") -> ("错误输出"=w389:errorcluster, "新路径"=w385:path)  [unwired: 9 in]
        n180 = call <vilib>:"Create Report.vi"("report type"=Report_Type."Excel", "template (empty)"=w385, "error in (no error)"=w389) -> ("report out"=w395:refnum<class "NI_report.lvclass">, "error out"=w391:errorcluster)  [unwired: 11 in]
        n181 = call-poly <vilib>:"Append Table to Report.vi"("report in"=w395, "column width (1)"=0.5, "column headers"=w393, "row headers"=w392, "numerical data"=w394, "error in (no error)"=w391) -> ("report out"=w386:refnum<class "NI_report.lvclass">, "error out"=w388:errorcluster)  [unwired: 6 in, 2 out]
        n182 = call-dynamic "Save Report to File.vi"("report in"=w386, "report file path"=w385, "error in (no error)"=w388) -> ("error out"=w387:errorcluster)  [unwired: 11 in, 1 out]
        n183 = call <vilib>:"Clear Errors.vi"("error in (no error)"=w387) -> ()  [unwired: 5 in, 2 out]
      }
      frame "loadT1" {
        n184 = call "文件对话框"() -> ("selected path"=w415:path, "error out"=w413:errorcluster)  [unwired: 12 in, 2 out]
        n185 = call "读取Excel至多列列表框.vi"("error in (no error)"=w413, "Excel表格路径"=w415) -> ("error out"=w412:errorcluster, "混响数值"=w409:string[][], "列首"=w411:string[], "行首"=w410:string[])  [unwired: 6 in]
        n186 = call "Enqueue Message (Single).vi"("error in (no error)"=w406, "消息"="safe", "消息队列"=w407) -> ("error out"=w404:cluster{"状态":bool, "代码":i32, "源":string}, "消息队列副本"=w405:refnum<queue>)  [unwired: 7 in]
        n187 = property class="MCListbox (严格)"(reference=w414, error in=w412, "ItemNames"=w409, "RowHdrs[]"=w410, "ColHdrString"=w411) -> ()  [unwired: 2 out]
      }
      frame "loadT2" {
        n188 = call "文件对话框2"() -> ("selected path"=w427:path, "error out"=w426:errorcluster)  [unwired: 12 in, 2 out]
        n189 = call "读取Excel至多列列表框.vi"("error in (no error)"=w426, "Excel表格路径"=w427) -> ("error out"=w425:errorcluster, "混响数值"=w422:string[][], "列首"=w424:string[], "行首"=w423:string[])  [unwired: 6 in]
        n190 = call "Enqueue Message (Single).vi"("error in (no error)"=w417, "消息"="safe", "消息队列"=w418) -> ("error out"=w419:cluster{"状态":bool, "代码":i32, "源":string}, "消息队列副本"=w420:refnum<queue>)  [unwired: 7 in]
        n191 = property class="MCListbox (严格)"(reference=w416, error in=w425, "ItemNames"=w422, "RowHdrs[]"=w423, "ColHdrString"=w424) -> ()  [unwired: 2 out]
      }
      frame "ExcelT2" {
        n192 = property class="MCListbox (严格)"(reference=w441) -> ("ItemNames"=w446:string[][], "RowHdrs[]"=w430:string[], "ColHdrString"=w431:string[])  [unwired: 1 in, 2 out]
        n193 = call "每列有效平均值.vi"("测试数组"=w446) -> ("混响2D数值"=w429:dbl[][])  [unwired: 9 in, 1 out]
        n194 = call "Enqueue Message (Single).vi"("error in (no error)"=w445, "消息"="safe", "消息队列"=w444) -> ("error out"=w442:cluster{"状态":bool, "代码":i32, "源":string}, "消息队列副本"=w443:refnum<queue>)  [unwired: 7 in]
        n195 = call "复制模板路径.vi"("名称前缀"="放样后测试_") -> ("错误输出"=w436:errorcluster, "新路径"=w432:path)  [unwired: 9 in]
        n196 = call <vilib>:"Create Report.vi"("report type"=Report_Type."Excel", "template (empty)"=w432, "error in (no error)"=w436) -> ("report out"=w439:refnum<class "NI_report.lvclass">, "error out"=w438:errorcluster)  [unwired: 11 in]
        n197 = call-poly <vilib>:"Append Table to Report.vi"("report in"=w439, "column width (1)"=0.5, "column headers"=w431, "row headers"=w430, "numerical data"=w429, "error in (no error)"=w438) -> ("report out"=w433:refnum<class "NI_report.lvclass">, "error out"=w435:errorcluster)  [unwired: 6 in, 2 out]
        n198 = call-dynamic "Save Report to File.vi"("report in"=w433, "report file path"=w432, "error in (no error)"=w435) -> ("error out"=w434:errorcluster)  [unwired: 11 in, 1 out]
        n199 = call <vilib>:"Clear Errors.vi"("error in (no error)"=w434) -> ()  [unwired: 5 in, 2 out]
      }
      frame "ExcelAllResult" {
        n200 = property class="MCListbox (严格)"(reference=w462) -> (error out=w449:errorcluster, "ItemNames"=w450:string[][], "RowHdrs[]"=w451:string[], "ColHdrString"=w452:string[])  [unwired: 1 in, 1 out]
        n201 = call "Enqueue Message (Single).vi"("error in (no error)"=w463, "消息"="safe", "消息队列"=w464) -> ()  [unwired: 7 in, 2 out]
        n202 = call "复制模板路径.vi"("错误输入"=w449, "名称前缀"="所有结果_") -> ("错误输出"=w457:errorcluster, "新路径"=w453:path)  [unwired: 8 in]
        n203 = call <vilib>:"Create Report.vi"("report type"=Report_Type."Excel", "template (empty)"=w453, "error in (no error)"=w457) -> ("report out"=w460:refnum<class "NI_report.lvclass">, "error out"=w459:errorcluster)  [unwired: 11 in]
        n204 = call-poly <vilib>:"Append Table to Report.vi"("report in"=w460, "column width (1)"=0.5, "column headers"=w452, "row headers"=w451, "text data"=w450, "error in (no error)"=w459) -> ("report out"=w454:refnum<class "NI_report.lvclass">, "error out"=w456:errorcluster)  [unwired: 6 in, 2 out]
        n205 = call-dynamic "Save Report to File.vi"("report in"=w454, "report file path"=w453, "error in (no error)"=w456) -> ("error out"=w455:errorcluster)  [unwired: 11 in, 1 out]
        n206 = call <vilib>:"Clear Errors.vi"("error in (no error)"=w455) -> ()  [unwired: 5 in, 2 out]
      }
      frame "ExportReport" {
        n207 = property class="MCListbox (严格)"(reference=w476) -> ("ItemNames"=w486:string[][], "RowHdrs[]"=w481:string[], "ColHdrString"=w482:string[])  [unwired: 1 in, 2 out]
        n208 = call "每列有效平均值.vi"("测试数组"=w486) -> ("混响2D数值"=w483:dbl[][])  [unwired: 9 in, 1 out]
        n209 = call "Enqueue Message (Single).vi"("error in (no error)"=w477, "消息"="safe", "消息队列"=w478) -> ()  [unwired: 7 in, 2 out]
        n210 = call "复制模板路径.vi"("名称前缀"="测试报告_") -> ("错误输出"=w470:errorcluster, "新路径"=w466:path)  [unwired: 9 in]
        n211 = call <vilib>:"Create Report.vi"("report type"=Report_Type."Excel", "template (empty)"=w466, "error in (no error)"=w470) -> ("report out"=w484:refnum<class "NI_report.lvclass">, "error out"=w480:errorcluster)  [unwired: 11 in]
        n212 = call-poly <vilib>:"Append Table to Report.vi"("report in"=w484, "column width (1)"=0.5, "column headers"=w482, "row headers"=w481, "numerical data"=w483, "error in (no error)"=w480) -> ("report out"=w474:refnum<class "NI_report.lvclass">, "error out"=w473:errorcluster)  [unwired: 6 in, 2 out]
        n213 = call-dynamic "Append Control Image to Report.vi"("report in"=w474, "ctrl reference"=w472, "error in (no error)"=w473, "MS Office parameters"=T23 {"position (Excel)"={"row"=10, "column"=0}, "name (Excel)"="", "bookmark (Word)"=""}) -> ("report out"=w469:refnum<class "NI_report.lvclass">, "error out"=w468:errorcluster)  [unwired: 8 in, 2 out]
        n214 = call-dynamic "Save Report to File.vi"("report in"=w469, "report file path"=w466, "error in (no error)"=w468) -> ("error out"=w467:errorcluster)  [unwired: 11 in, 1 out]
        n215 = call <vilib>:"Clear Errors.vi"("error in (no error)"=w467) -> ()  [unwired: 5 in, 2 out]
      }
      frame "Exti" {
        n216 = Flush Queue(queue=w491, error in (no error)=w489) -> (queue out=w490:refnum<queue>, error out=w488:errorcluster)  [unwired: 1 out]
      }
    }
  }
  n217 = while {
    tunnel: w22 -> [w502]
    shift-right: [w500] -> w40
    shift-left: w43 -> [w501]
    tunnel: w13 -> [w499]
    tunnel: w10 -> [w498]
    tunnel: w9 -> [w497]
    tunnel: w8 -> [w496]
    tunnel: w3 -> [w495]
    tunnel: w2 -> [w494]
    tunnel: w1 -> [w493]
    stop <- w503 stop-if-true
    # "事件处理"
    n218 = event shown="[22] \"测试类型\": 值改变" {
      selector: w501 -> [_ _ _ _ _ _ _ _ _ _ _ _ _ _ _ _ _ _ _ _ _ _ _ _ _ _ _ _ _ _ _ _ _ _]
      dyn-events: [_ _ _ _ _ _ _ _ _ _ _ _ _ _ _ _ _ _ _ _ _ _ _ _ _ _ _ _ _ _ _ _ _ _] -> w500
      timeout: _ -> [_ _ _ _ _ _ _ _ _ _ _ _ _ _ _ _ _ _ _ _ _ _ _ _ _ _ _ _ _ _ _ _ _ _]
      tunnel: [_ w507 _ _ _ _ _ _ TRUE _ _ _ _ _ _ _ _ _ _ _ _ _ _ _ _ _ _ _ _ _ _ _ _ _] -> w503
      tunnel: w502 -> [_ w504 w509 w510 w512 w515 w516 w519 _ w522 w524 w526 w528 w530 w532 w534 _ _ _ _ _ _ _ w598 w600 w602 w604 w606 w608 w610 _ _ _ w621]
      tunnel: w499 -> [_ _ _ _ _ _ _ _ _ _ _ _ _ _ _ _ w536 w538 w540 w542 _ _ w579 _ _ _ _ _ _ _ _ _ _ _]
      tunnel: w498 -> [_ _ _ _ _ _ _ _ _ _ _ _ _ _ _ _ _ _ _ _ _ _ w576 _ _ _ _ _ _ _ w612 _ _ _]
      tunnel: w497 -> [_ _ _ _ _ _ _ _ _ _ _ _ _ _ _ _ _ _ _ _ _ _ w578 _ _ _ _ _ _ _ _ w617 _ _]
      tunnel: w496 -> [_ _ _ _ _ _ _ _ _ _ _ _ _ _ _ _ _ _ _ _ _ _ w577 _ _ _ _ _ _ _ _ _ w620 _]
      tunnel: w495 -> [_ _ _ _ _ _ _ _ _ _ _ _ _ _ _ _ _ _ _ _ w556 w572 _ _ _ _ _ _ _ _ _ _ _ _]
      tunnel: w494 -> [_ _ _ _ _ _ _ _ _ _ _ _ _ _ _ _ _ _ _ _ _ w562 _ _ _ _ _ _ _ _ _ _ _ _]
      tunnel: w493 -> [_ _ _ _ _ _ _ _ _ _ _ _ _ _ _ _ _ _ _ _ w552 _ _ _ _ _ _ _ _ _ _ _ _ _]
      event Timeout {
        n219 = event-data() -> ()  [unwired: 1 in, 3 out]
      }
      event Panel Close? {
        w507 = TRUE ("放弃？")
        n220 = event-data() -> ()  [unwired: 1 in, 4 out]
        n221 = call "Enqueue Message (Single).vi"("优先消息？ (F)"=TRUE, "消息"="Exti", "消息队列"=w504) -> ()  [unwired: 7 in, 2 out]
        n222 = event-data("Discard?"=w507) -> ()  [unwired: 1 in, 1 out]
      }
      event Value Change {
        n223 = event-data() -> ()  [unwired: 1 in, 1 out]
        n224 = call "Enqueue Message (Single).vi"("消息"="HWsetup", "消息队列"=w509) -> ()  [unwired: 8 in, 2 out]
      }
      event Value Change {
        n225 = event-data() -> ()  [unwired: 1 in, 1 out]
        n226 = call "Enqueue Message (Single).vi"("消息"="EMsetup", "消息队列"=w510) -> ()  [unwired: 8 in, 2 out]
      }
      event Value Change {
        n227 = event-data() -> ()  [unwired: 1 in, 1 out]
        n228 = call "Enqueue Message (Single).vi"("消息"="calibration", "消息队列"=w512) -> ()  [unwired: 8 in, 2 out]
      }
      event Value Change {
        n229 = event-data() -> ()  [unwired: 1 in, 1 out]
        n230 = call "Enqueue Message (Single).vi"("消息"="start", "消息队列"=w515) -> ()  [unwired: 8 in, 2 out]
      }
      event Value Change {
        n231 = event-data() -> ()  [unwired: 1 in, 1 out]
        n232 = call "Enqueue Message (Single).vi"("消息"="stop", "消息队列"=w516) -> ()  [unwired: 8 in, 2 out]
      }
      event Value Change {
        n233 = event-data() -> ()  [unwired: 1 in, 1 out]
        n234 = call "Enqueue Message (Single).vi"("优先消息？ (F)"=TRUE, "消息"="Exti", "消息队列"=w519) -> ()  [unwired: 7 in, 2 out]
      }
      event User Event {
        n235 = event-data() -> ()  [unwired: 1 in, 1 out]
      }
      event Value Change {
        n236 = event-data() -> ()  [unwired: 1 in, 1 out]
        n237 = call "Enqueue Message (Single).vi"("消息"="saveT1", "消息队列"=w522) -> ()  [unwired: 8 in, 2 out]
      }
      event Value Change {
        n238 = event-data() -> ()  [unwired: 1 in, 1 out]
        n239 = call "Enqueue Message (Single).vi"("消息"="saveT2", "消息队列"=w524) -> ()  [unwired: 8 in, 2 out]
      }
      event "deletelineT1": Value Change {
        n240 = event-data() -> ()  [unwired: 1 in, 1 out]
        n241 = call "Enqueue Message (Single).vi"("消息"="deletelineT1", "消息队列"=w526) -> ()  [unwired: 8 in, 2 out]
      }
      event "deletelineT2": Value Change {
        n242 = event-data() -> ()  [unwired: 1 in, 1 out]
        n243 = call "Enqueue Message (Single).vi"("消息"="deletelineT2", "消息队列"=w528) -> ()  [unwired: 8 in, 2 out]
      }
      event "clearlistT1": Value Change {
        n244 = event-data() -> ()  [unwired: 1 in, 1 out]
        n245 = call "Enqueue Message (Single).vi"("消息"="clearlistT1", "消息队列"=w530) -> ()  [unwired: 8 in, 2 out]
      }
      event "clearlistT2": Value Change {
        n246 = event-data() -> ()  [unwired: 1 in, 1 out]
        n247 = call "Enqueue Message (Single).vi"("消息"="clearlistT2", "消息队列"=w532) -> ()  [unwired: 8 in, 2 out]
      }
      event Value Change {
        n248 = event-data() -> ()  [unwired: 1 in, 1 out]
        n249 = call "Enqueue Message (Single).vi"("消息"="analysis", "消息队列"=w534) -> ()  [unwired: 8 in, 2 out]
      }
      event Value Change {
        n250 = event-data() -> ()  [unwired: 1 in, 1 out]
        n251 = property class="TabCtl (严格)"(reference=w536, "Value"=T10."空场测试结果" ("值")) -> ()  [unwired: 1 in, 2 out]
      }
      event Value Change {
        n252 = event-data() -> ()  [unwired: 1 in, 1 out]
        n253 = property class="TabCtl (严格)"(reference=w538, "Value"=T10."放入样品后测试结果" ("值")) -> ()  [unwired: 1 in, 2 out]
      }
      event "返回空场测试": Value Change {
        n254 = event-data() -> ()  [unwired: 1 in, 1 out]
        n255 = property class="TabCtl (严格)"(reference=w540, "Value"=T10."空场当前结果" ("值")) -> ()  [unwired: 1 in, 2 out]
      }
      event "返回放样后测试": Value Change {
        n256 = event-data() -> ()  [unwired: 1 in, 1 out]
        n257 = property class="TabCtl (严格)"(reference=w542, "Value"=T10."放入样品后当前结果" ("值")) -> ()  [unwired: 1 in, 2 out]
      }
      event Value Change {
        # "关时颜色\n开时颜色"
        n258 = event-data() -> ("NewVal"=w551:T12)  [unwired: 1 in]
        n259 = Unbundle By Name(w556) -> ("空场当前结果"=w555:refnum<vi>, "放样后当前结果"=w554:refnum<vi>, "分析结果"=w545:refnum<vi>, "导出报告"=w544:refnum<vi>)
        n260 = Select(t=cluster{u32, u32}[] [{4424887, 9134235}, {4424887, 9134235}, {4424887, 4424887}, {4424887, 4424887}, {4424887, 16777216}, {16777216, 16777216}] ("颜色[4]"), s=w551, f=cluster{u32, u32}[] [{16777216, 16777216}, {4424887, 4424887}, {4424887, 4424887}, {4424887, 4424887}, {4424887, 16777216}, {16777216, 16777216}] ("颜色[4]")) -> (s? t:f=w559:cluster{u32, u32}[])
        n261 = property class="Bool (严格)"(reference=w552) -> ("Value"=w550:bool)  [unwired: 1 in, 2 out]
        n262 = Select(t=T25."Enabled" ("禁用"), s=w551, f=T25."Disabled and Grayed Out" ("禁用")) -> (s? t:f=w553:T25)
        n263 = And(x=w551, y=w550) -> (x .and. y?=w547:T12)
        n264 = property class="Bool (严格)"(reference=w555, "Colors [4]"=w559) -> ()  [unwired: 1 in, 2 out]
        n265 = Select(t=T25."Enabled" ("禁用"), s=w547, f=T25."Disabled and Grayed Out" ("禁用")) -> (s? t:f=w546:T25)
        n266 = property class="Bool (严格)"(reference=w554, "DisabledEnum"=w553) -> ()  [unwired: 1 in, 2 out]
        n267 = property class="Bool (严格)"(reference=w545, "DisabledEnum"=w546) -> ()  [unwired: 1 in, 2 out]
        n268 = property class="Bool (严格)"(reference=w544, "DisabledEnum"=w546) -> ()  [unwired: 1 in, 2 out]
      }
      event Value Change {
        n269 = event-data() -> ("NewVal"=w568:T12)  [unwired: 1 in]
        n270 = Unbundle By Name(w572) -> ("放样后当前结果"=w571:refnum<vi>, "分析结果"=w570:refnum<vi>, "导出报告"=w569:refnum<vi>)
        n271 = property class="Bool (严格)"(reference=w562) -> ("Value"=w567:bool)  [unwired: 1 in, 2 out]
        n272 = And(x=w568, y=w567) -> (x .and. y?=w566:T12)
        n273 = Select(t=cluster{u32, u32}[] [{4424887, 9134235}, {4424887, 9134235}, {4424887, 4424887}, {4424887, 4424887}, {4424887, 4424887}, {4424887, 4424887}] ("颜色[4]"), s=w568, f=cluster{u32, u32}[] [{16777216, 16777216}, {4424887, 4424887}, {4424887, 4424887}, {4424887, 4424887}, {4424887, 4424887}, {16777216, 16777216}] ("颜色[4]")) -> (s? t:f=w573:cluster{u32, u32}[])
        n274 = Select(t=T25."Enabled" ("禁用"), s=w566, f=T25."Disabled and Grayed Out" ("禁用")) -> (s? t:f=w563:T25)
        n275 = property class="Bool (严格)"(reference=w571, "Colors [4]"=w573) -> ()  [unwired: 1 in, 2 out]
        n276 = property class="Bool (严格)"(reference=w570, "DisabledEnum"=w563) -> ()  [unwired: 1 in, 2 out]
        n277 = property class="Bool (严格)"(reference=w569, "DisabledEnum"=w563) -> ()  [unwired: 1 in, 2 out]
      }
      event "测试类型": Value Change {
        n278 = event-data() -> ("NewVal"=w581:enum32{"空场当前结果", "放样后当前结果", "分析结果", "导出报告"})  [unwired: 1 in]
        n279 = case shown="\"导出报告\"" w581 {
          tunnel: [T10."空场当前结果" ("值") T10."放入样品后当前结果" ("值") T10."分析结果" ("值") T10."分析结果" ("值")] -> w580
          tunnel: w578 -> [w584 _ w590 w594]
          tunnel: w577 -> [w582 w586 _ _]
          tunnel: w576 -> [_ w587 w591 w595]
          frame "空场当前结果", Default {
            w583 = FALSE ("可见")
            n280 = property class="Str (严格)"(reference=w584, "Visible"=w583) -> ()  [unwired: 1 in, 2 out]
            n281 = property class="Str (严格)"(reference=w582, "Visible"=w583) -> ()  [unwired: 1 in, 2 out]
          }
          frame "放样后当前结果" {
            w588 = FALSE ("可见")
            n282 = property class="Str (严格)"(reference=w587, "Visible"=w588) -> ()  [unwired: 1 in, 2 out]
            n283 = property class="Str (严格)"(reference=w586, "Visible"=w588) -> ()  [unwired: 1 in, 2 out]
          }
          frame "分析结果" {
            w592 = FALSE ("可见")
            n284 = property class="Str (严格)"(reference=w591, "Visible"=w592) -> ()  [unwired: 1 in, 2 out]
            n285 = property class="Str (严格)"(reference=w590, "Visible"=w592) -> ()  [unwired: 1 in, 2 out]
          }
          frame "导出报告" {
            w596 = FALSE ("可见")
            n286 = property class="Str (严格)"(reference=w595, "Visible"=w596) -> ()  [unwired: 1 in, 2 out]
            n287 = property class="Str (严格)"(reference=w594, "Visible"=w596) -> ()  [unwired: 1 in, 2 out]
          }
        }
        n288 = property class="TabCtl (严格)"(reference=w579, "Value"=w580) -> ()  [unwired: 1 in, 2 out]
      }
      event "空场结果至Excel": Value Change {
        n289 = event-data() -> ()  [unwired: 1 in, 1 out]
        n290 = call "Enqueue Message (Single).vi"("消息"="ExcelT1", "消息队列"=w598) -> ()  [unwired: 8 in, 2 out]
      }
      event "放样结果至Excel": Value Change {
        n291 = event-data() -> ()  [unwired: 1 in, 1 out]
        n292 = call "Enqueue Message (Single).vi"("消息"="ExcelT2", "消息队列"=w600) -> ()  [unwired: 8 in, 2 out]
      }
      event Value Change {
        n293 = event-data() -> ()  [unwired: 1 in, 1 out]
        n294 = call "Enqueue Message (Single).vi"("消息"="ExcelAllResult", "消息队列"=w602) -> ()  [unwired: 8 in, 2 out]
      }
      event Value Change {
        n295 = event-data() -> ()  [unwired: 1 in, 1 out]
        n296 = call "Enqueue Message (Single).vi"("消息"="ExportReport", "消息队列"=w604) -> ()  [unwired: 8 in, 2 out]
      }
      event "loadT1": Value Change {
        n297 = event-data() -> ()  [unwired: 1 in, 1 out]
        n298 = call "Enqueue Message (Single).vi"("消息"="loadT1", "消息队列"=w606) -> ()  [unwired: 8 in, 2 out]
      }
      event "loadT2": Value Change {
        n299 = event-data() -> ()  [unwired: 1 in, 1 out]
        n300 = call "Enqueue Message (Single).vi"("消息"="loadT2", "消息队列"=w608) -> ()  [unwired: 8 in, 2 out]
      }
      event Value Change {
        n301 = event-data() -> ()  [unwired: 1 in, 1 out]
        n302 = call "Enqueue Message (Single).vi"("消息"="NewMeasurement", "消息队列"=w610) -> ()  [unwired: 8 in, 2 out]
      }
      event "空场混响频谱图": Mouse Move {
        n303 = event-data() -> ("CtlRef"=w614:refnum<vi>, "Coords"=w613:T26)  [unwired: 1 in]
        n304 = call "鼠标获取曲线值.vi"("鼠标坐标"=w613, "图谱引用"=w614, "字符引用"=w612) -> ()  [unwired: 9 in]
      }
      event "放入样品后混响频谱图": Mouse Move {
        n305 = event-data() -> ("CtlRef"=w616:refnum<vi>, "Coords"=w615:T26)  [unwired: 1 in]
        n306 = call "鼠标获取曲线值.vi"("鼠标坐标"=w615, "图谱引用"=w616, "字符引用"=w617) -> ()  [unwired: 9 in]
      }
      event "吸声频谱图": Mouse Move {
        n307 = event-data() -> ("CtlRef"=w619:refnum<vi>, "Coords"=w618:T26)  [unwired: 1 in]
        n308 = call "鼠标获取曲线值.vi"("鼠标坐标"=w618, "图谱引用"=w619, "字符引用"=w620) -> ()  [unwired: 9 in]
      }
      event Menu Selection (User) {
        n309 = event-data() -> ("ItemTag"=w622:string)  [unwired: 1 in]
        n310 = case shown="\"关于\"" w622 {
          tunnel: w621 -> [_ w623 w625 _ _ _ _ w632 w634 w636 w638 _]
          frame "假", Default {
          }
          frame "新的测量" {
            n311 = call "Enqueue Message (Single).vi"("消息"="NewMeasurement", "消息队列"=w623) -> ()  [unwired: 8 in, 2 out]
          }
          frame "退出" {
            n312 = call "Enqueue Message (Single).vi"("优先消息？ (F)"=TRUE, "消息"="Exti", "消息队列"=w625) -> ()  [unwired: 7 in, 2 out]
          }
          frame "通道1" {
            w628 = enum16{"通道1", "通道2", "通道3", "通道4"}."通道1" ("通道选择")
            n313 = call "SoundCalibration.vi"("通道号"=w628, "通道选择"=w628) -> ()  [unwired: 10 in]
          }
          frame "通道2" {
            w629 = enum16{"通道1", "通道2", "通道3", "通道4"}."通道2" ("通道选择")
            n314 = call "SoundCalibration.vi"("通道号"=w629, "通道选择"=w629) -> ()  [unwired: 10 in]
          }
          frame "通道3" {
            w630 = enum16{"通道1", "通道2", "通道3", "通道4"}."通道3" ("通道选择")
            n315 = call "SoundCalibration.vi"("通道号"=w630, "通道选择"=w630) -> ()  [unwired: 10 in]
          }
          frame "通道4" {
            w631 = enum16{"通道1", "通道2", "通道3", "通道4"}."通道4" ("通道选择")
            n316 = call "SoundCalibration.vi"("通道号"=w631, "通道选择"=w631) -> ()  [unwired: 10 in]
          }
          frame "硬件设置" {
            n317 = call "Enqueue Message (Single).vi"("消息"="HWsetup", "消息队列"=w632) -> ()  [unwired: 8 in, 2 out]
          }
          frame "环境参数设置" {
            n318 = call "Enqueue Message (Single).vi"("消息"="EMsetup", "消息队列"=w634) -> ()  [unwired: 8 in, 2 out]
          }
          frame "开始" {
            n319 = call "Enqueue Message (Single).vi"("消息"="start", "消息队列"=w636) -> ()  [unwired: 8 in, 2 out]
          }
          frame "停止" {
            n320 = call "Enqueue Message (Single).vi"("消息"="stop", "消息队列"=w638) -> ()  [unwired: 8 in, 2 out]
          }
          frame "关于" {
            n321 = One Button Dialog(message="斯万泰科\n958A\n四通道数据采集仪" ("消息")) -> ()  [unwired: 1 in, 1 out]
          }
        }
      }
    }
  }
  n322 = while {
    tunnel: w22 -> [w653]
    tunnel: w41 -> [w651]
    tunnel: w37 -> [w649]
    tunnel: [w648] -> w36
    tunnel: w35 -> [w645]
    tunnel: w24 -> [w644]
    tunnel: w2 -> [w643]
    tunnel: w1 -> [w642]
    tunnel: w3 -> [w641]
    stop <- w650 stop-if-true
    # "消息处理"
    n323 = call "Dequeue Message.vi"("error in (no error)"=w649, "消息队列"=w653) -> ("error out"=w646:cluster{"状态":bool, "代码":i32, "源":string}, "消息"=w652:string, "消息队列副本"=w647:refnum<queue>)  [unwired: 6 in, 1 out]
    n324 = case shown="\"Initialize\"" w652 {
      tunnel: w651 -> [_ _ _ _ _ _ _ _ _ _ _ _ _ _ _ _ _ _ _ _ _ w804]
      tunnel: [_ _ _ _ _ _ _ _ _ _ _ _ _ _ _ _ _ _ _ _ _ TRUE] -> w650
      tunnel: [w654 w666 w670 w677 _ w688 w691 w698 _ w711 _ w724 w734 w738 w745 w752 w761 w766 w773 w781 w787 w802] -> w648
      tunnel: w647 -> [_ w668 w673 w680 _ w689 w694 w701 w707 w714 w720 w726 w732 w739 w748 w755 w762 w769 w776 w780 w794 w796]
      tunnel: w646 -> [w654 w667 w672 w678 _ w686 w692 w699 w705 w712 w719 w725 w733 w740 w746 w753 w759 w767 w774 w782 _ _]
      tunnel: w645 -> [_ _ w671 w679 _ w687 w693 _ _ _ _ _ _ _ _ _ _ _ _ _ w792 w801]
      tunnel: w644 -> [_ _ _ _ _ _ _ w700 w706 w713 w718 w727 w731 w741 w747 w754 w760 w768 w775 w783 w790 w799]
      tunnel: w643 -> [_ w664 _ _ _ _ _ _ _ _ _ _ _ _ _ _ _ _ _ _ _ _]
      tunnel: w642 -> [_ w663 _ _ _ _ _ _ _ _ _ _ _ _ _ _ _ _ _ _ _ _]
      tunnel: w641 -> [_ w661 _ _ _ _ _ _ _ _ _ _ _ _ _ _ _ _ _ _ _ _]
      frame "safe", Default {
        n325 = Wait (ms)(milliseconds to wait=u32 20 ("等待时间（毫秒）")) -> ()  [unwired: 1 out]
      }
      frame "Initialize" {
        w656 = T25."Disabled and Grayed Out" ("禁用")
        w662 = FALSE
        w665 = cluster{u32, u32}[] [{16777216, 16777216}, {4424887, 4424887}, {4424887, 4424887}, {4424887, 4424887}, {4424887, 16777216}, {16777216, 16777216}] ("颜色[4]")
        # "颜色和页面恢复初始"
        n326 = Unbundle By Name(w661) -> ("空场当前结果"=w660:refnum<vi>, "放样后当前结果"=w659:refnum<vi>, "分析结果"=w658:refnum<vi>, "导出报告"=w657:refnum<vi>)
        n327 = property class="Bool (严格)"(reference=w664, "Value"=w662) -> ()  [unwired: 1 in, 2 out]
        n328 = property class="Bool (严格)"(reference=w663, "Value"=w662) -> ()  [unwired: 1 in, 2 out]
        n329 = call "Enqueue Message (Single).vi"("error in (no error)"=w667, "消息"="safe", "消息队列"=w668) -> ("error out"=w666:cluster{"状态":bool, "代码":i32, "源":string})  [unwired: 7 in, 1 out]
        n330 = property class="Bool (严格)"(reference=w660, "Colors [4]"=w665) -> ()  [unwired: 1 in, 2 out]
        n331 = property class="Bool (严格)"(reference=w659, "Colors [4]"=w665, "DisabledEnum"=w656) -> ()  [unwired: 1 in, 2 out]
        n332 = property class="Bool (严格)"(reference=w658, "DisabledEnum"=w656) -> ()  [unwired: 1 in, 2 out]
        n333 = property class="Bool (严格)"(reference=w657, "DisabledEnum"=w656) -> ()  [unwired: 1 in, 2 out]
      }
      frame "calibration" {
        n334 = call "Enqueue Message (Single).vi"("error in (no error)"=w672, "消息"="safe", "消息队列"=w673) -> ("error out"=w674:cluster{"状态":bool, "代码":i32, "源":string})  [unwired: 7 in, 1 out]
        n335 = call "Enqueue Message (Single).vi"("error in (no error)"=w674, "消息"="calibration", "消息队列"=w671) -> ("error out"=w670:cluster{"状态":bool, "代码":i32, "源":string})  [unwired: 7 in, 1 out]
      }
      frame "HWsetup" {
        n336 = call "Enqueue Message (Single).vi"("error in (no error)"=w678, "消息"="HWsetup", "消息队列"=w679) -> ("error out"=w682:cluster{"状态":bool, "代码":i32, "源":string})  [unwired: 7 in, 1 out]
        n337 = call "Enqueue Message (Single).vi"("error in (no error)"=w682, "消息"="safe", "消息队列"=w680) -> ("error out"=w677:cluster{"状态":bool, "代码":i32, "源":string})  [unwired: 7 in, 1 out]
      }
      frame "EMsetup" {
        n338 = call "EMsetup options.vi"() -> ()  [unwired: 12 in]
      }
      frame "start" {
        n339 = call "Enqueue Message (Single).vi"("error in (no error)"=w686, "消息"="start", "消息队列"=w687) -> ("error out"=w685:cluster{"状态":bool, "代码":i32, "源":string})  [unwired: 7 in, 1 out]
        n340 = call "Enqueue Message (Single).vi"("error in (no error)"=w685, "消息"="safe", "消息队列"=w689) -> ("error out"=w688:cluster{"状态":bool, "代码":i32, "源":string})  [unwired: 7 in, 1 out]
      }
      frame "stop" {
        n341 = call "Enqueue Message (Single).vi"("error in (no error)"=w692, "消息"="stop", "消息队列"=w693) -> ("error out"=w696:cluster{"状态":bool, "代码":i32, "源":string})  [unwired: 7 in, 1 out]
        n342 = call "Enqueue Message (Single).vi"("error in (no error)"=w696, "消息"="safe", "消息队列"=w694) -> ("error out"=w691:cluster{"状态":bool, "代码":i32, "源":string})  [unwired: 7 in, 1 out]
      }
      frame "saveT1" {
        n343 = call "Enqueue Message (Single).vi"("error in (no error)"=w699, "消息"="saveT1", "消息队列"=w700) -> ("error out"=w703:cluster{"状态":bool, "代码":i32, "源":string})  [unwired: 7 in, 1 out]
        n344 = call "Enqueue Message (Single).vi"("error in (no error)"=w703, "消息"="safe", "消息队列"=w701) -> ("error out"=w698:cluster{"状态":bool, "代码":i32, "源":string})  [unwired: 7 in, 1 out]
      }
      frame "saveT2" {
        n345 = call "Enqueue Message (Single).vi"("error in (no error)"=w705, "消息"="saveT2", "消息队列"=w706) -> ("error out"=w710:cluster{"状态":bool, "代码":i32, "源":string})  [unwired: 7 in, 1 out]
        n346 = call "Enqueue Message (Single).vi"("error in (no error)"=w710, "消息"="safe", "消息队列"=w707) -> ()  [unwired: 7 in, 2 out]
      }
      frame "deletelineT1" {
        n347 = call "Enqueue Message (Single).vi"("error in (no error)"=w712, "消息"="deletelineT1", "消息队列"=w713) -> ("error out"=w717:cluster{"状态":bool, "代码":i32, "源":string})  [unwired: 7 in, 1 out]
        n348 = call "Enqueue Message (Single).vi"("error in (no error)"=w717, "消息"="safe", "消息队列"=w714) -> ("error out"=w711:cluster{"状态":bool, "代码":i32, "源":string})  [unwired: 7 in, 1 out]
      }
      frame "deletelineT2" {
        n349 = call "Enqueue Message (Single).vi"("error in (no error)"=w719, "消息"="deletelineT2", "消息队列"=w718) -> ("error out"=w723:cluster{"状态":bool, "代码":i32, "源":string})  [unwired: 7 in, 1 out]
        n350 = call "Enqueue Message (Single).vi"("error in (no error)"=w723, "消息"="safe", "消息队列"=w720) -> ()  [unwired: 7 in, 2 out]
      }
      frame "clearlistT1" {
        n351 = call "Enqueue Message (Single).vi"("error in (no error)"=w725, "消息"="clearlistT1", "消息队列"=w727) -> ("error out"=w730:cluster{"状态":bool, "代码":i32, "源":string})  [unwired: 7 in, 1 out]
        n352 = call "Enqueue Message (Single).vi"("error in (no error)"=w730, "消息"="safe", "消息队列"=w726) -> ("error out"=w724:cluster{"状态":bool, "代码":i32, "源":string})  [unwired: 7 in, 1 out]
      }
      frame "clearlistT2" {
        n353 = call "Enqueue Message (Single).vi"("error in (no error)"=w733, "消息"="clearlistT2", "消息队列"=w731) -> ("error out"=w737:cluster{"状态":bool, "代码":i32, "源":string})  [unwired: 7 in, 1 out]
        n354 = call "Enqueue Message (Single).vi"("error in (no error)"=w737, "消息"="safe", "消息队列"=w732) -> ("error out"=w734:cluster{"状态":bool, "代码":i32, "源":string})  [unwired: 7 in, 1 out]
      }
      frame "analysis" {
        n355 = call "Enqueue Message (Single).vi"("error in (no error)"=w740, "消息"="analysis", "消息队列"=w741) -> ("error out"=w744:cluster{"状态":bool, "代码":i32, "源":string})  [unwired: 7 in, 1 out]
        n356 = call "Enqueue Message (Single).vi"("error in (no error)"=w744, "消息"="safe", "消息队列"=w739) -> ("error out"=w738:cluster{"状态":bool, "代码":i32, "源":string})  [unwired: 7 in, 1 out]
      }
      frame "ExcelT1" {
        n357 = call "Enqueue Message (Single).vi"("error in (no error)"=w746, "消息"="ExcelT1", "消息队列"=w747) -> ("error out"=w751:cluster{"状态":bool, "代码":i32, "源":string})  [unwired: 7 in, 1 out]
        n358 = call "Enqueue Message (Single).vi"("error in (no error)"=w751, "消息"="safe", "消息队列"=w748) -> ("error out"=w745:cluster{"状态":bool, "代码":i32, "源":string})  [unwired: 7 in, 1 out]
      }
      frame "loadT1" {
        n359 = call "Enqueue Message (Single).vi"("error in (no error)"=w753, "消息"="loadT1", "消息队列"=w754) -> ("error out"=w758:cluster{"状态":bool, "代码":i32, "源":string})  [unwired: 7 in, 1 out]
        n360 = call "Enqueue Message (Single).vi"("error in (no error)"=w758, "消息"="safe", "消息队列"=w755) -> ("error out"=w752:cluster{"状态":bool, "代码":i32, "源":string})  [unwired: 7 in, 1 out]
      }
      frame "loadT2" {
        n361 = call "Enqueue Message (Single).vi"("error in (no error)"=w759, "消息"="loadT2", "消息队列"=w760) -> ("error out"=w765:cluster{"状态":bool, "代码":i32, "源":string})  [unwired: 7 in, 1 out]
        n362 = call "Enqueue Message (Single).vi"("error in (no error)"=w765, "消息"="safe", "消息队列"=w762) -> ("error out"=w761:cluster{"状态":bool, "代码":i32, "源":string})  [unwired: 7 in, 1 out]
      }
      frame "ExcelT2" {
        n363 = call "Enqueue Message (Single).vi"("error in (no error)"=w767, "消息"="ExcelT2", "消息队列"=w768) -> ("error out"=w772:cluster{"状态":bool, "代码":i32, "源":string})  [unwired: 7 in, 1 out]
        n364 = call "Enqueue Message (Single).vi"("error in (no error)"=w772, "消息"="safe", "消息队列"=w769) -> ("error out"=w766:cluster{"状态":bool, "代码":i32, "源":string})  [unwired: 7 in, 1 out]
      }
      frame "ExcelAllResult" {
        n365 = call "Enqueue Message (Single).vi"("error in (no error)"=w774, "消息"="ExcelAllResult", "消息队列"=w775) -> ("error out"=w779:cluster{"状态":bool, "代码":i32, "源":string})  [unwired: 7 in, 1 out]
        n366 = call "Enqueue Message (Single).vi"("error in (no error)"=w779, "消息"="safe", "消息队列"=w776) -> ("error out"=w773:cluster{"状态":bool, "代码":i32, "源":string})  [unwired: 7 in, 1 out]
      }
      frame "ExportReport" {
        n367 = call "Enqueue Message (Single).vi"("error in (no error)"=w782, "消息"="ExportReport", "消息队列"=w783) -> ("error out"=w786:cluster{"状态":bool, "代码":i32, "源":string})  [unwired: 7 in, 1 out]
        n368 = call "Enqueue Message (Single).vi"("error in (no error)"=w786, "消息"="safe", "消息队列"=w780) -> ("error out"=w781:cluster{"状态":bool, "代码":i32, "源":string})  [unwired: 7 in, 1 out]
      }
      frame "NewMeasurement" {
        n369 = call "Enqueue Message (Single).vi"("消息"="Initialize", "消息队列"=w794) -> ("error out"=w789:cluster{"状态":bool, "代码":i32, "源":string})  [unwired: 8 in, 1 out]
        n370 = call "Enqueue Message (Single).vi"("error in (no error)"=w789, "消息"="reInitialize", "消息队列"=w792) -> ("error out"=w788:cluster{"状态":bool, "代码":i32, "源":string})  [unwired: 7 in, 1 out]
        n371 = call "Enqueue Message (Single).vi"("error in (no error)"=w788, "消息"="Initialize", "消息队列"=w790) -> ("error out"=w787:cluster{"状态":bool, "代码":i32, "源":string})  [unwired: 7 in, 1 out]
      }
      frame "Exti" {
        w797 = "Exti" ("消息")
        n372 = call "Enqueue Message (Single).vi"("优先消息？ (F)"=TRUE, "消息"=w797, "消息队列"=w801) -> ()  [unwired: 7 in, 2 out]
        n373 = call "Enqueue Message (Single).vi"("优先消息？ (F)"=TRUE, "消息"=w797, "消息队列"=w799) -> ()  [unwired: 7 in, 2 out]
        n374 = call "Fire User Event - Stop.vi"("用户事件－停止"=w804) -> ("error out"=w802:cluster{"状态":bool, "代码":i32, "源":string})  [unwired: 10 in]
        n375 = Flush Queue(queue=w796) -> ()  [unwired: 1 in, 3 out]
      }
    }
  }
  n376 = Release Queue(queue=w22, error in (no error)=w36) -> (error out=w32:errorcluster)  [unwired: 1 in, 2 out]
  n377 = Unregister For Events(event registration refnum=w40) -> (error out=w33:errorcluster)  [unwired: 1 in]
  n378 = Release Queue(queue=w31, error in (no error)=w27) -> (error out=w30:errorcluster)  [unwired: 1 in, 2 out]
  n379 = Release Queue(queue=w29, error in (no error)=w26) -> (error out=w28:errorcluster)  [unwired: 1 in, 2 out]
  n380 = Merge Errors(w33, w32, w30, w28) -> (w34:errorcluster)
  n381 = call "Destroy User Event - Stop.vi"("error in (no error)"=w34, "用户事件－停止"=w41) -> ()  [unwired: 9 in, 1 out]
